vi "Login Window Control.vi"() -> ()   [LabVIEW 2015]
uses:
  <vilib>/Utility/miscctls.llb/LVBoundsTypeDef.ctl
  <vilib>/Utility/miscctls.llb/LVPositionTypeDef.ctl
  EnumEstado.ctl
  Application/Type Ref. Notificacion Eventos.ctl
  Control 2.ctl
  Control 1.ctl
panel:
  in  "Stop Button":bool
  out "Tab Control 2":enum32{"MENU"}(tab)
  out "String":string
  in  "1":T1
  in  "Password":string
  in  "2":T1
  in  "3":T1
  in  "4":T1
  in  "5":T1
  in  "6":T1
  in  "7":T1
  in  "8":T1
  in  "9":T1
  in  "Log in":T1
  in  "Borrar":T1
  in  "Clear":T1
  out "Tab Control":T2(tab)
  in  "Tab1_Button_Temperatura_ambiente":bool
  in  "Tab1_Button_Temperatura_superficie":bool
  in  "Tab1_Button_Sinoptico":bool
  in  "logout":bool
  in  "Tab1_Button_Humedad":bool
  in  "Tab1_Button_Potencia":bool
  in  "Tab1_Button_Radiacion":bool
  out "Flujo_Bypass":bool
  out "Flujo_Load":bool
  out "Flujo_Bat_descarga":bool
  out "Flujo_Bat_carg":bool
  out "Flujo_Gen":bool
  out "Flujo_Panel":bool
  out "String 11":string
  out "String 10":string
  out "String 9":string
  out "String 8":string
  in  "Tab1_volver_sinoptico":bool
  out "Falla monofásica":bool caption="Falla \nmonofásica"
  out "Algun mal funcionamiento \nen el SGH":bool caption="Algun mal funcionamiento\nen el SGH"
  out "Alta temperatura\n en gabinete":bool caption="Alta temperatura en \ngabinete"
  out "Falla trifásica":bool caption="Falla\ntrifásica"
  out "Falla en módulo":bool
  out "valor_panel":dbl
  out "valor_carga":dbl
  out "valor_generador":dbl
  out "ÚLTIMA MEDICIÓN DEL\n G. DIESEL":timestamp
  out "ÚLTIMA MEDICIÓN DEL \nINVERSOR":timestamp
  out "valor_bateria":dbl
  out "Falla nivel de batería alta":bool caption="Falla nivel \nde\nbatería alta"
  out "Nivel de batería baja":bool caption="Nivel de\nbatería baja"
  out "Ring_Panel":u16(ring)
  out "Ring_Nivel_bat":u16(ring)
  out "Ring_Gen":u16(ring)
  out "Ring_Load":u16(ring)
  out "String 7":string
  out "Ring_Inversor":u16(ring)
  out "String 2":string
  in  "Radiacion Tab 1":bool
  in  "Tab1_volver_radiacion":bool
  out "Radiacion solar global":cluster{timestamp[], dbl[]}(graph)
  in  "Temperatura Tab 1":bool
  in  "Tab1_volver_tempambiente":bool
  out "XY Graph Temperatura":cluster{timestamp[], dbl[]}(graph)
  out "String 3":string
  in  "Tab1_volver_humedad":bool
  in  "Humedad Relativa Tab 1":bool
  out "XY Humedad Relativa":T3
  out "String 4":string
  in  "Temperatura de Panel Tab 1":bool
  in  "Tab1_volver_tempsuper":bool
  out "XY Graph Temperatura de Panel":cluster{timestamp[], dbl[]}(graph)
  out "String 5":string
  in  "Tab1_volver_potencia":bool
  in  "Pot_load_S Tab 1":bool
  in  "Pot_load_R Tab 1":bool
  in  "Potencia Panel Tab 1":bool
  in  "Pot_load_T Tab 1":bool
  in  "Pot_bat. Tab 1":bool
  in  "Pot_gen Tab 1":bool
  out "XY Graph Potencia":cluster{timestamp[], dbl[]}(graph)
  out "String 6":string
  # "SISTEMA DE MONITOREO PLANTA FOTOVOLTAICA \nMAYOR PABLO LAGERENZA"
  # "ACCESO"
  # "POTENCIA"
  # "ALMACENAMIENTO"
  # "SALIDA"
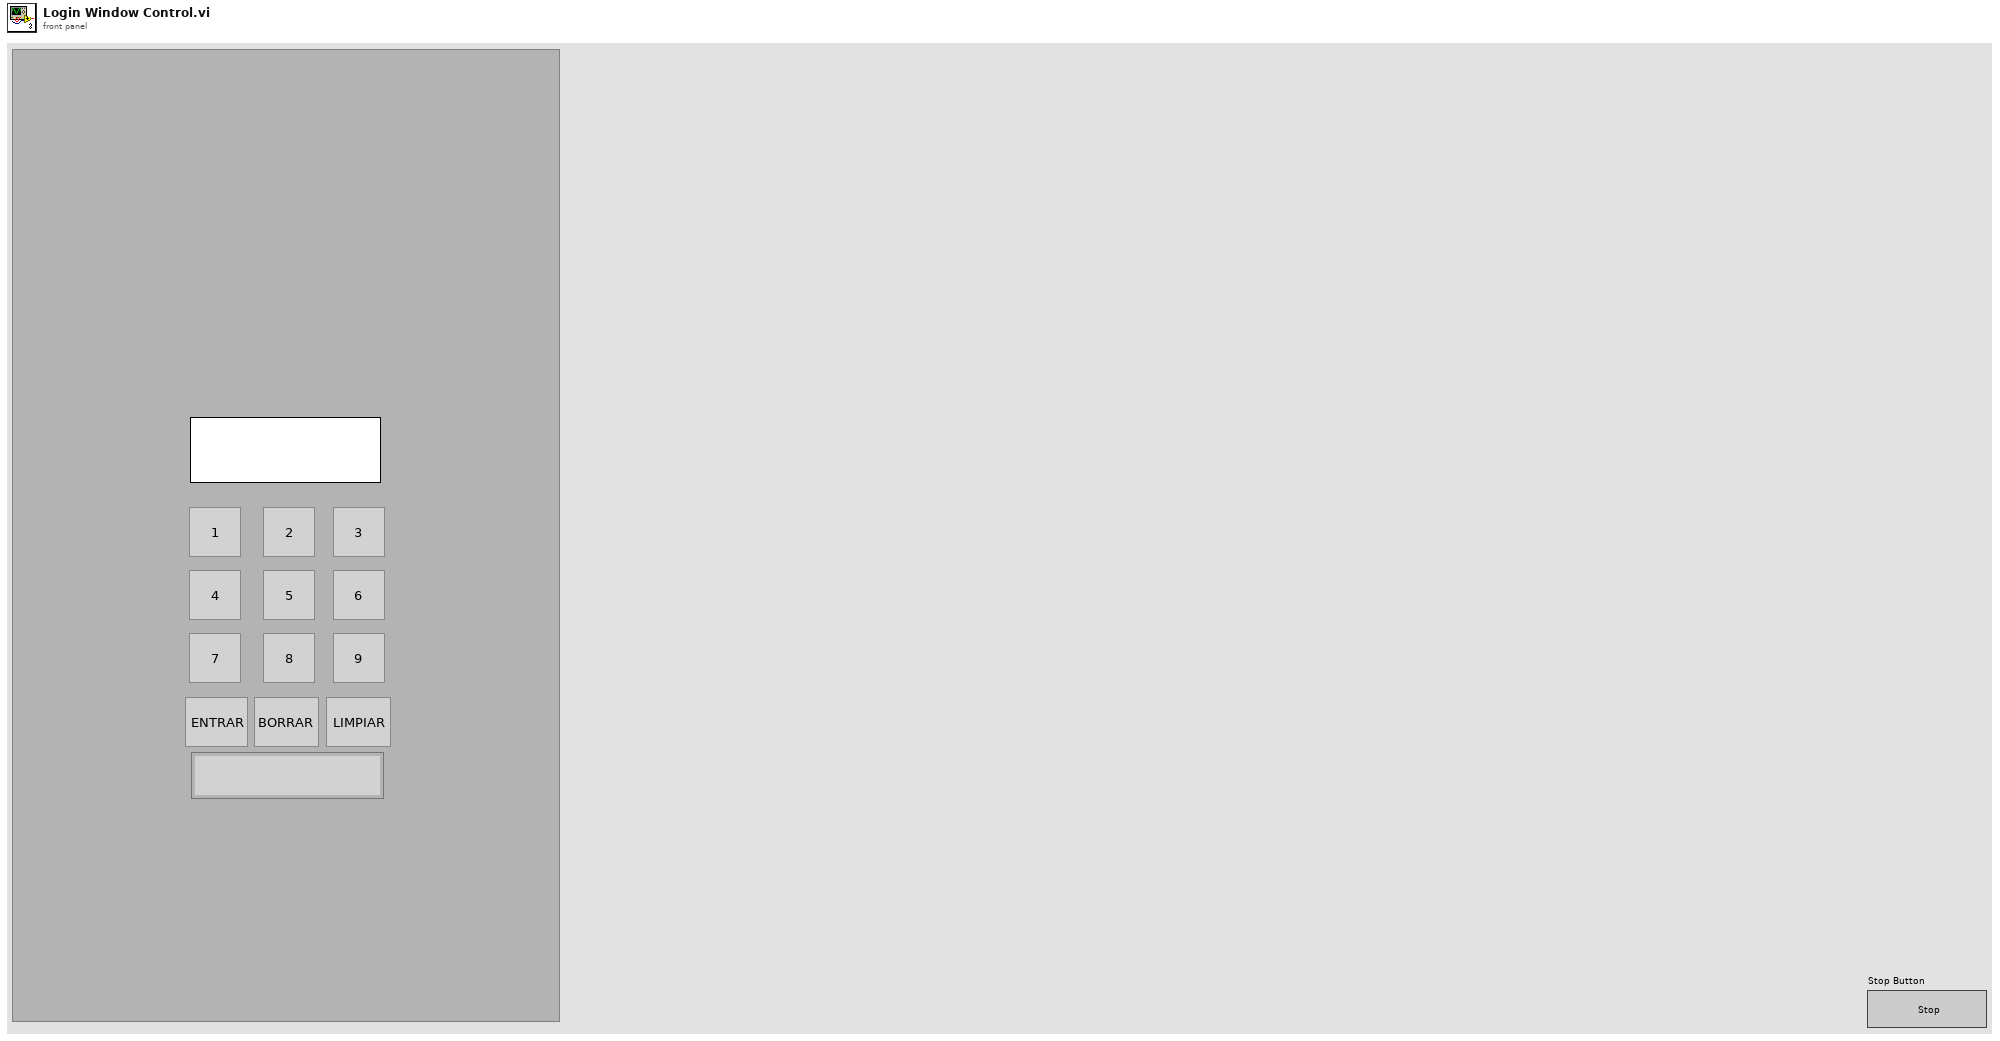
[diagram p1: front panel]
types:
  T1 = typedef "Control 2.ctl" = bool
  T2 = enum32{"MENU", "CUADRO SINOPTICO", "RADIACION SOLAR", "TEMPERATURA", "HUMEDAD RELATIVA", "TEMPERATURA DE SUPERFICIE", "POTENCIA"}
  T3 = typedef "Control 1.ctl" = cluster{timestamp[], dbl[]}
  T4 = typedef "LVPositionTypeDef.ctl" = cluster{"Left":i32, "Top":i32}
  T5 = typedef "LVBoundsTypeDef.ctl" = cluster{"Width":u32, "Height":u32}
  T6 = cluster{"queueM1 out":refnum<queue>, "queueM2 out":refnum<queue>, "queueM3 out":refnum<queue>}
  T7 = typedef "EnumEstado.ctl" = enum16{"Stop", "Iniciado", "Log In", "Log Out", "Escribir", "Leer Radiacion", "Leer Temp", "Leer Humed Relat", "Leer Temp del Panel", "Leer Pot Panel", "Leer Pot Fase R", "Leer Pot Fase  S", "Leer PotFase T", "Leer Nivel Bat", "Leer Pot Generador"}
  T8 = typedef "Type Ref. Notificacion Eventos.ctl" = enum32{"MENU", "CUADRO SINOPTICO", "RADIACION SOLAR", "TEMPERATURA", "HUMEDAD RELATIVA", "TEMPERATURA DE SUPERFICIE", "POTENCIA"}
  T9 = typedef "Semaphore RefNum" = refnum<k1>
  T10 = enum16{"open", "replace", "create", "open or create", "replace or create", "replace or create with confirmation"}
  T11 = cluster{"tdms control out":refnum<k34>, "tdms historial out":refnum<k34>, "tdms sinc out":refnum<k34>}
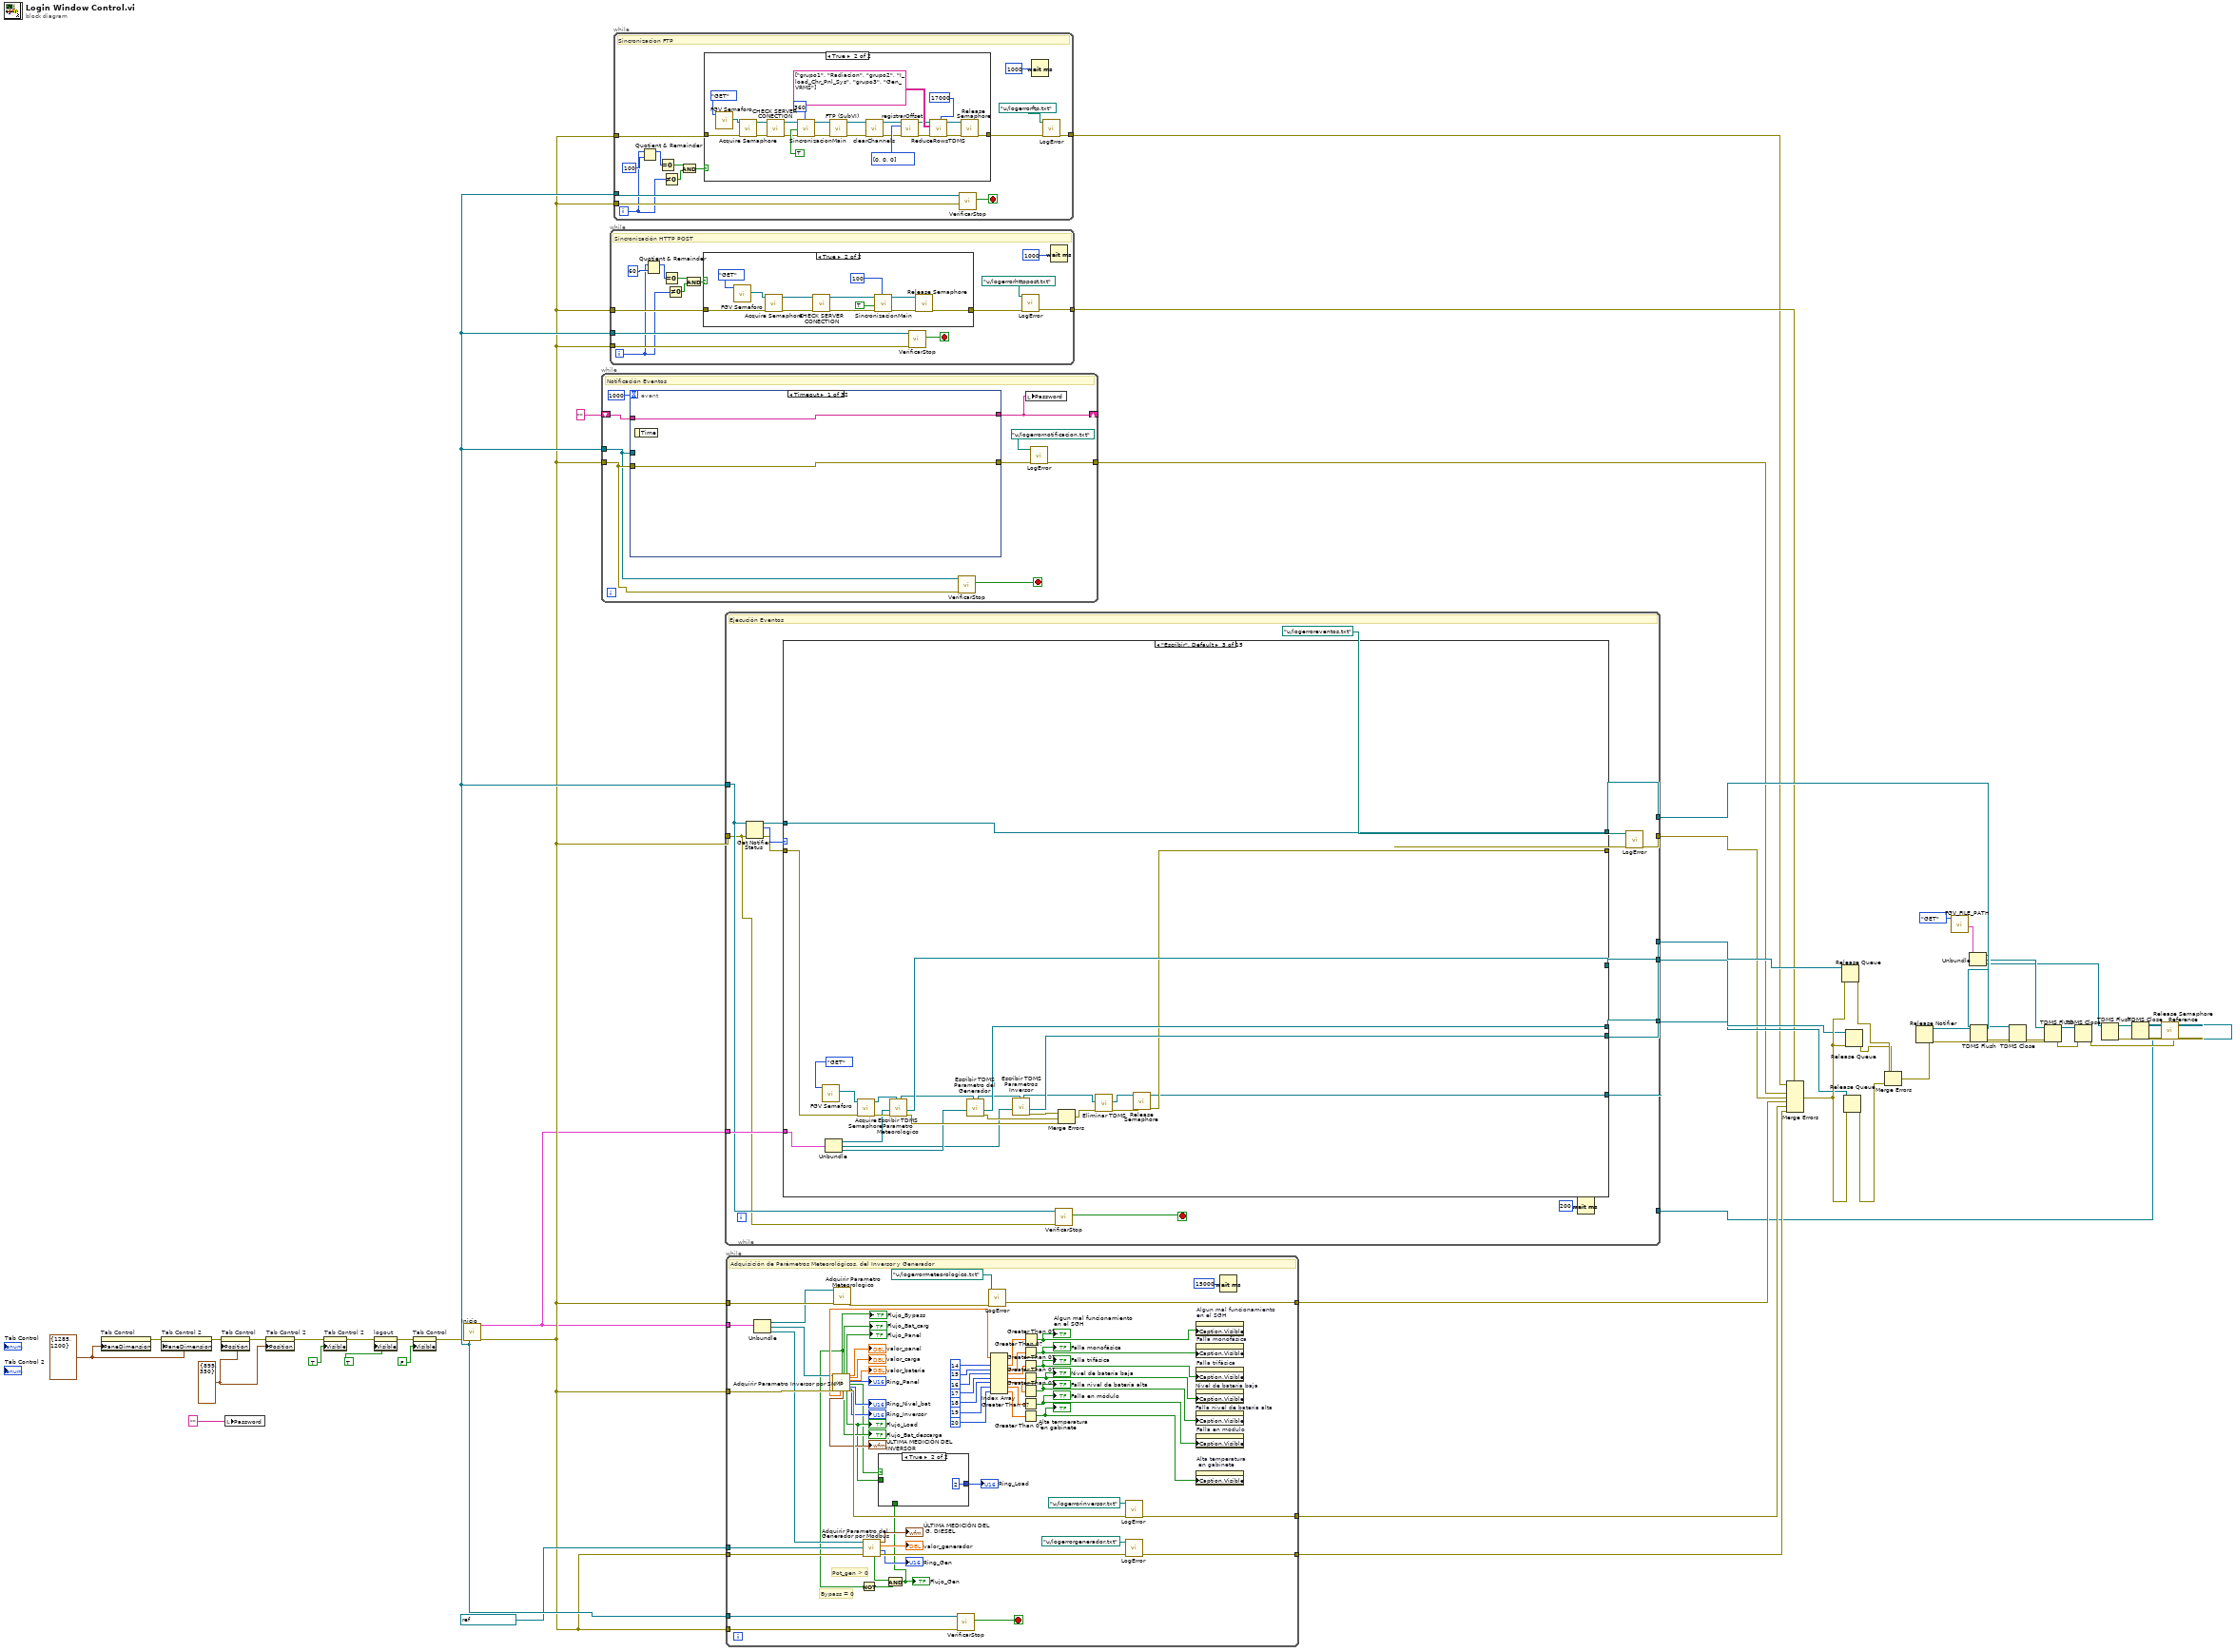
[diagram p0: block diagram]
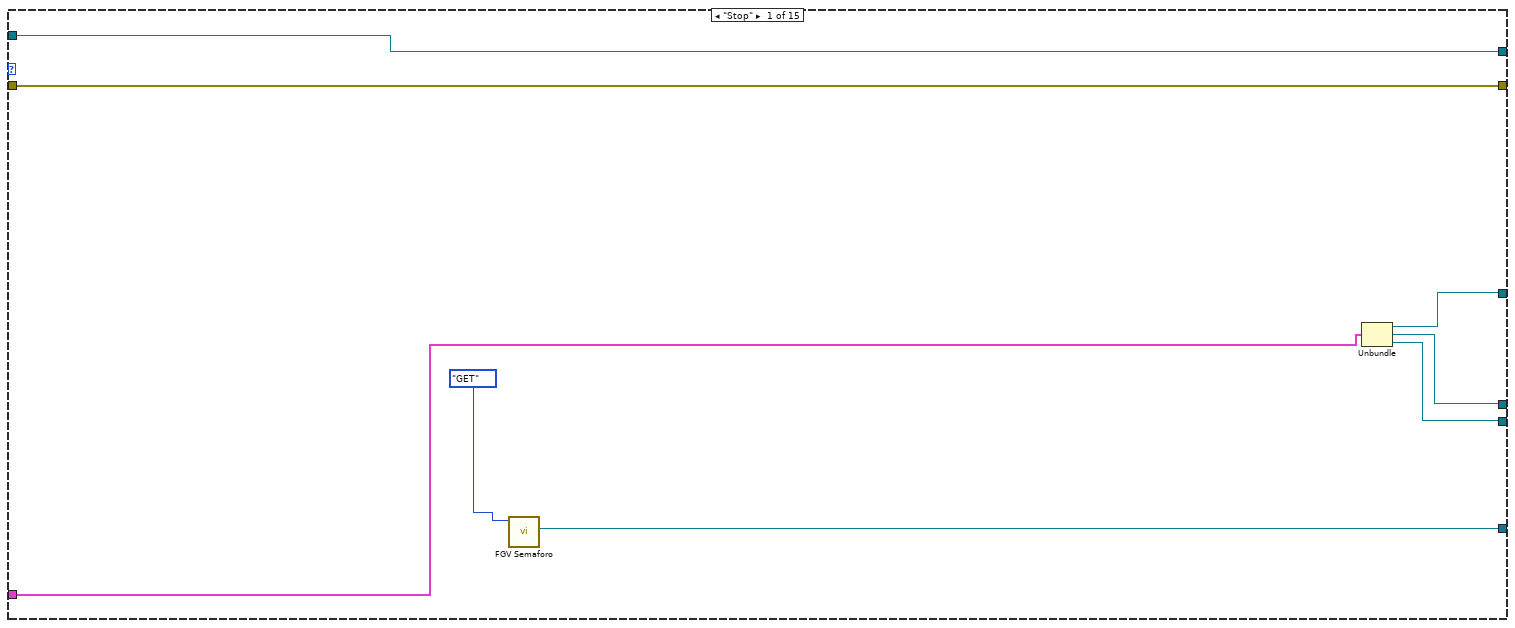
[diagram p4: hidden frame]
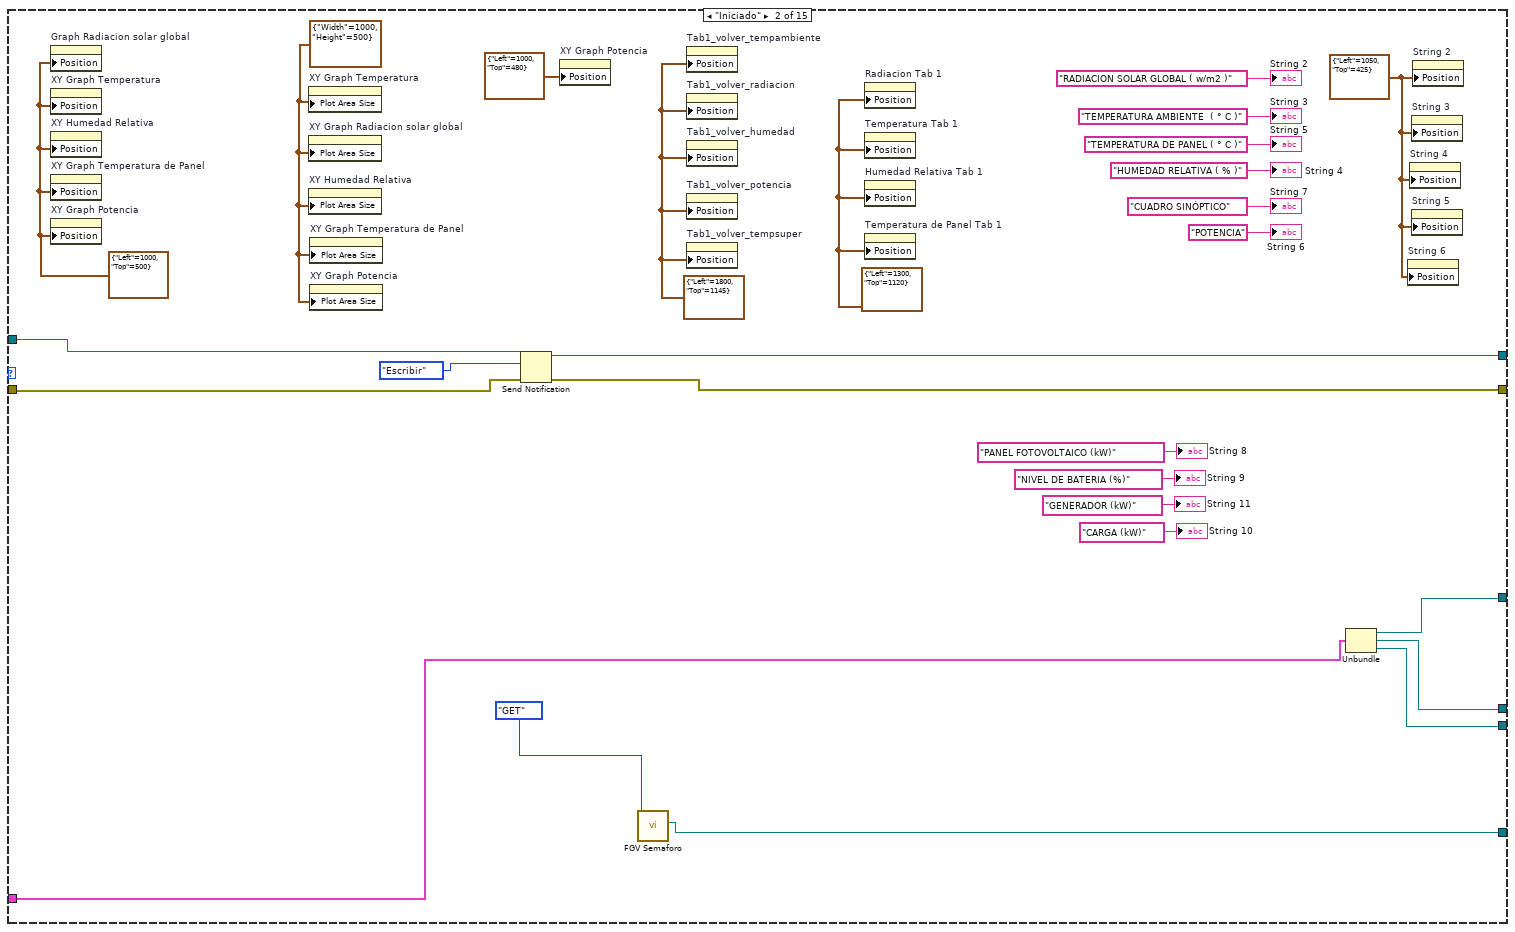
[diagram p5: hidden frame]
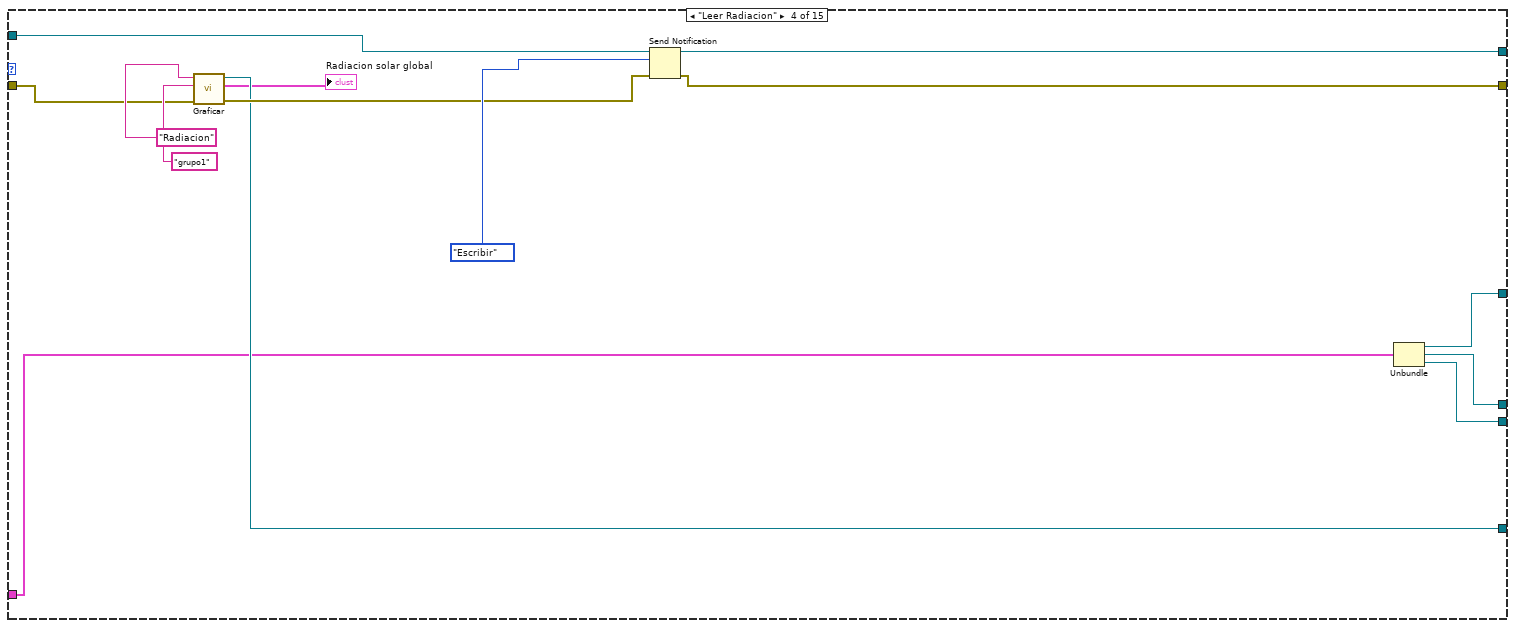
[diagram p6: hidden frame]
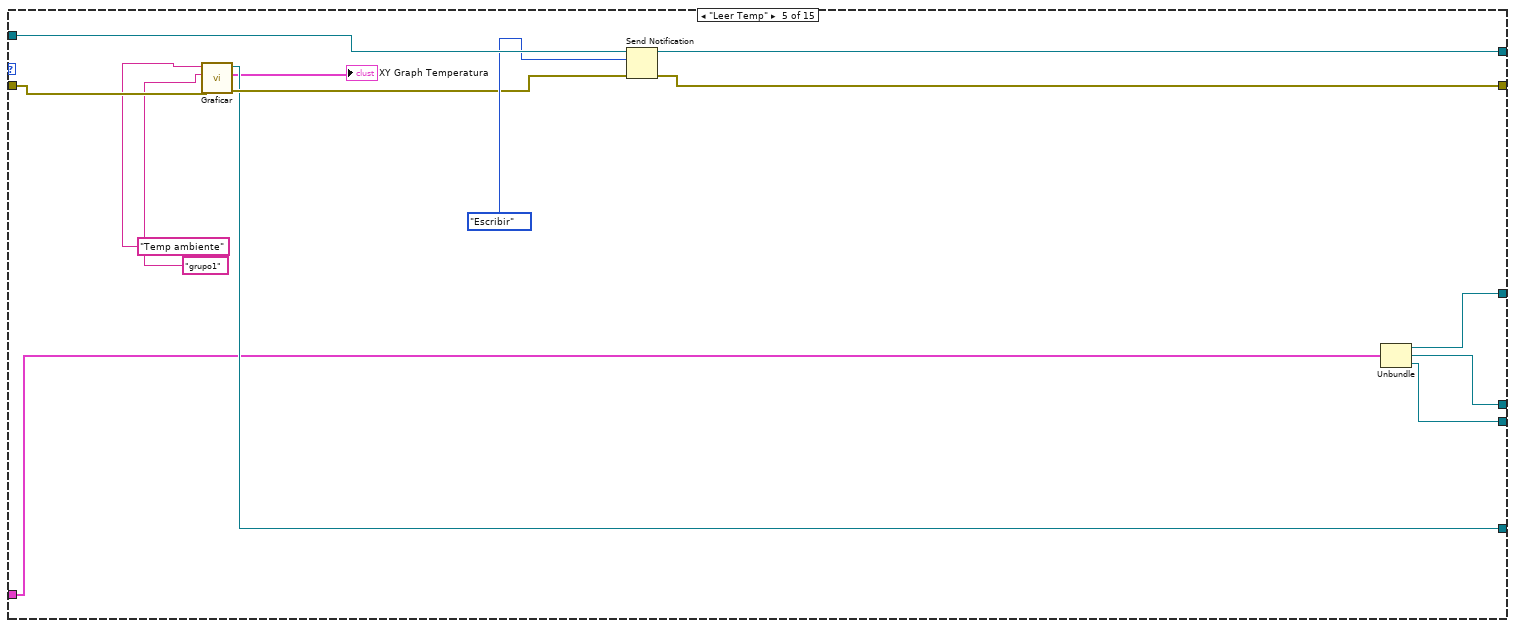
[diagram p7: hidden frame]
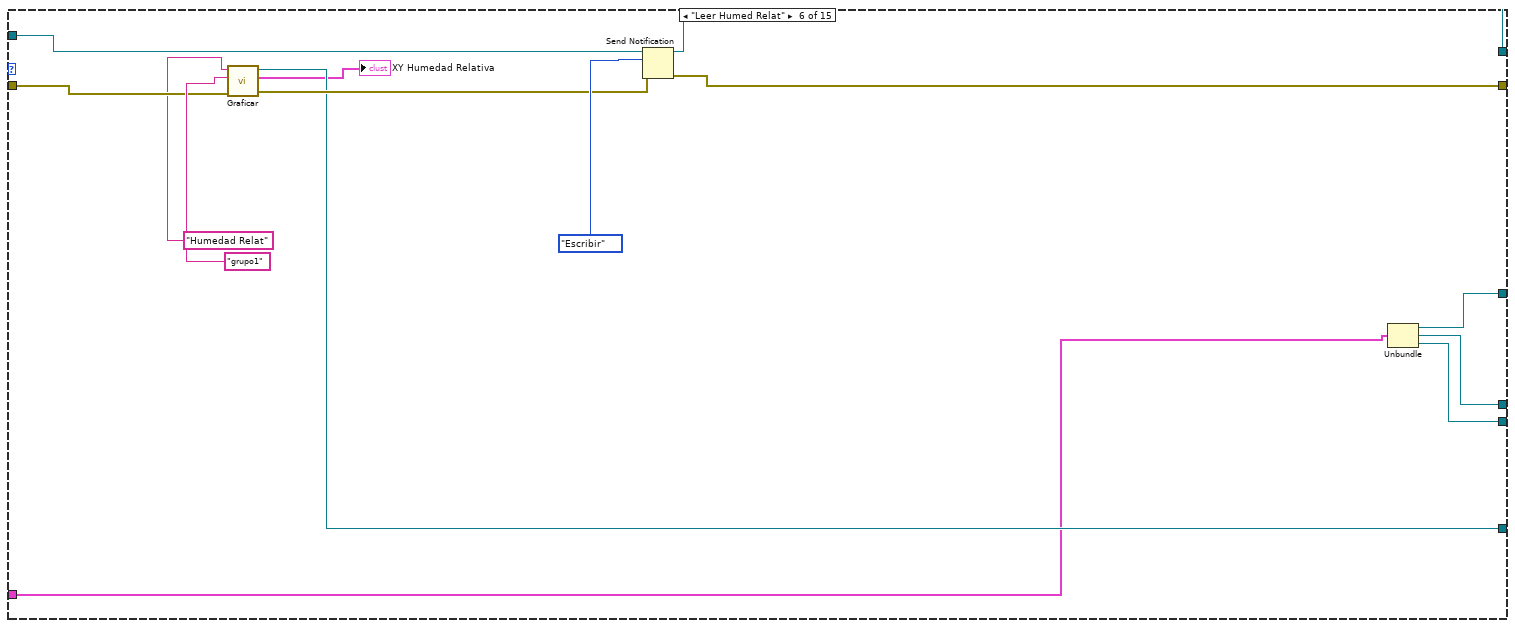
[diagram p8: hidden frame]
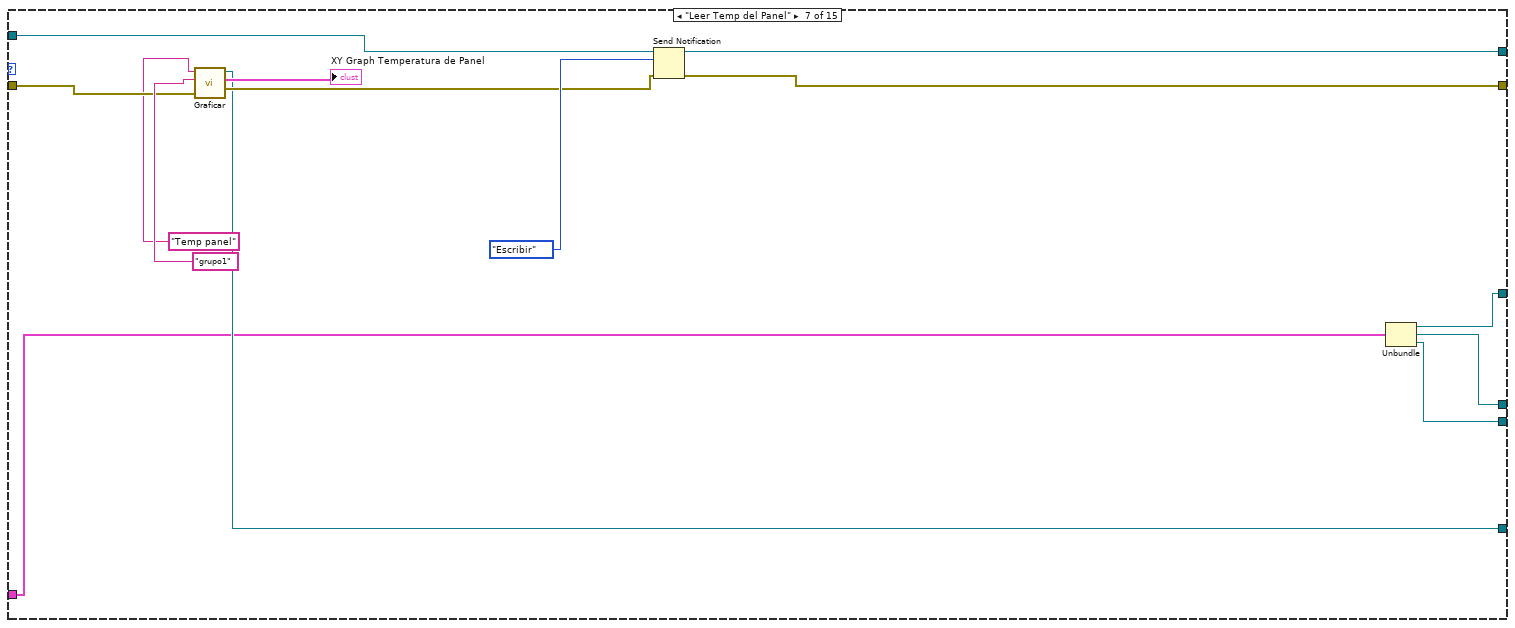
[diagram p9: hidden frame]
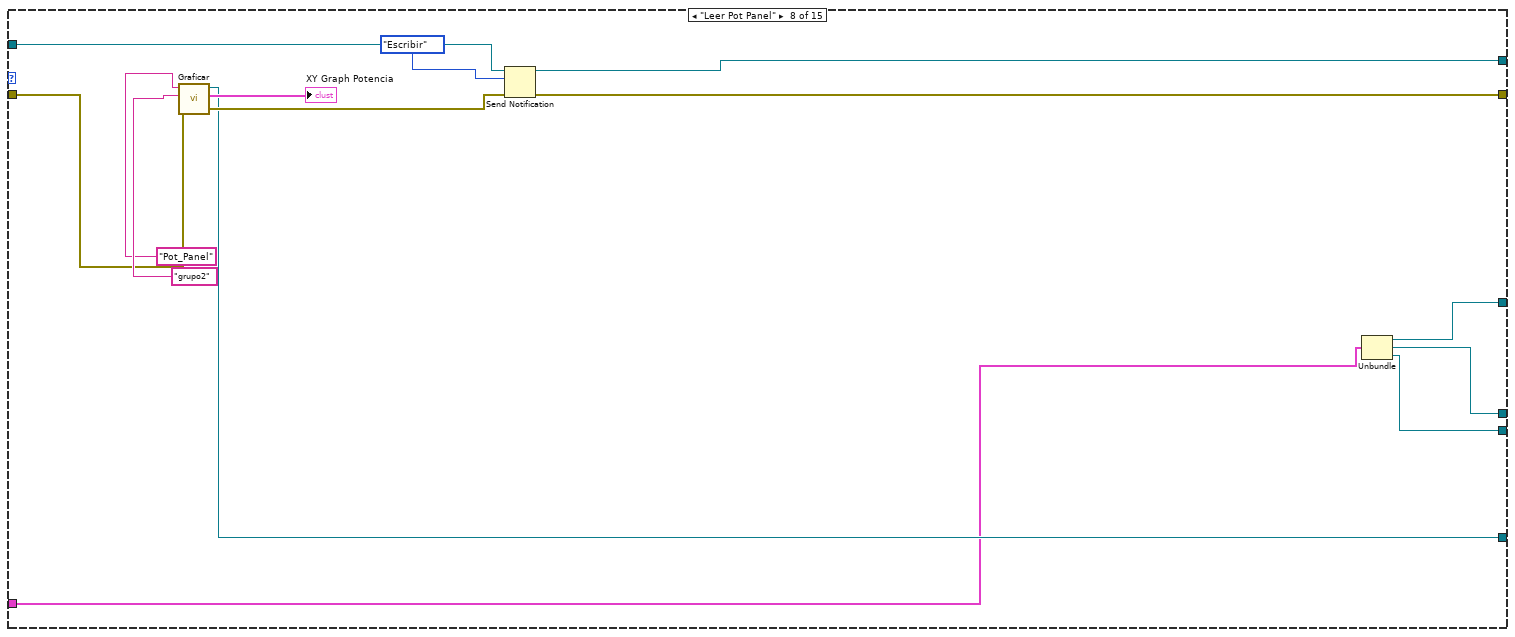
[diagram p10: hidden frame]
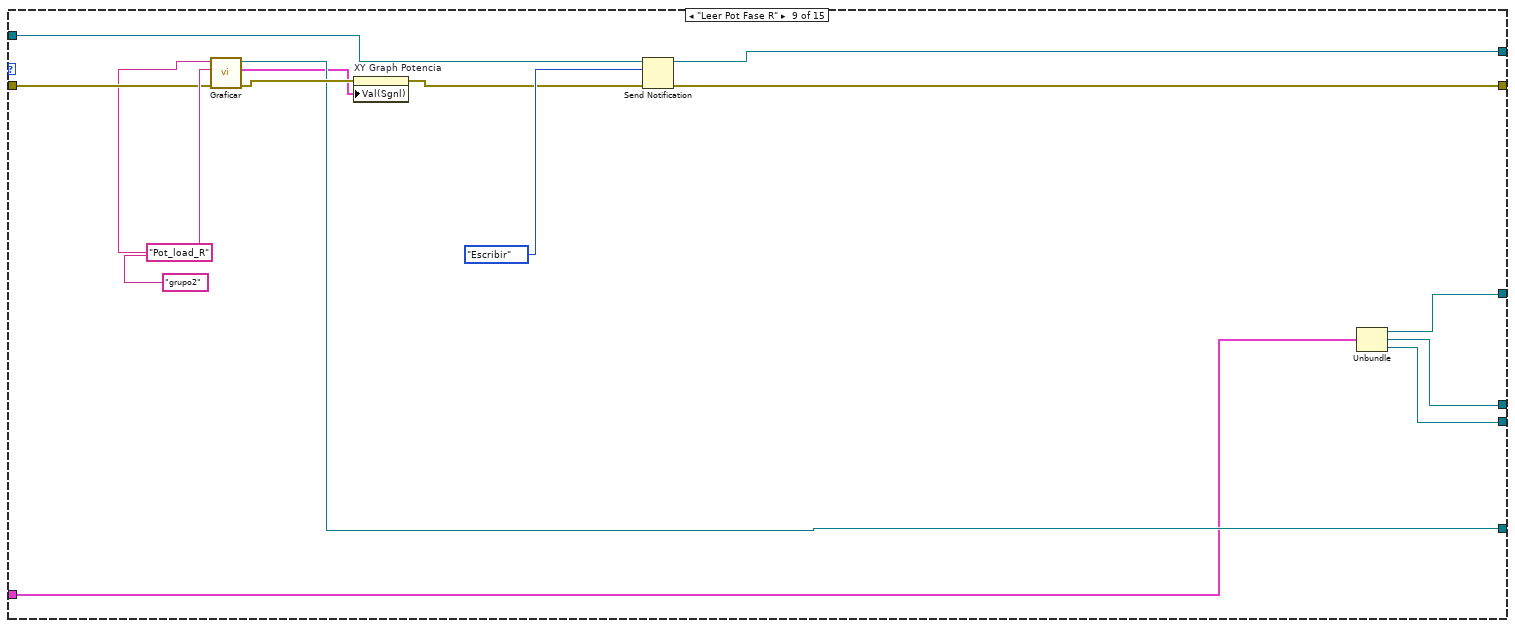
[diagram p11: hidden frame]
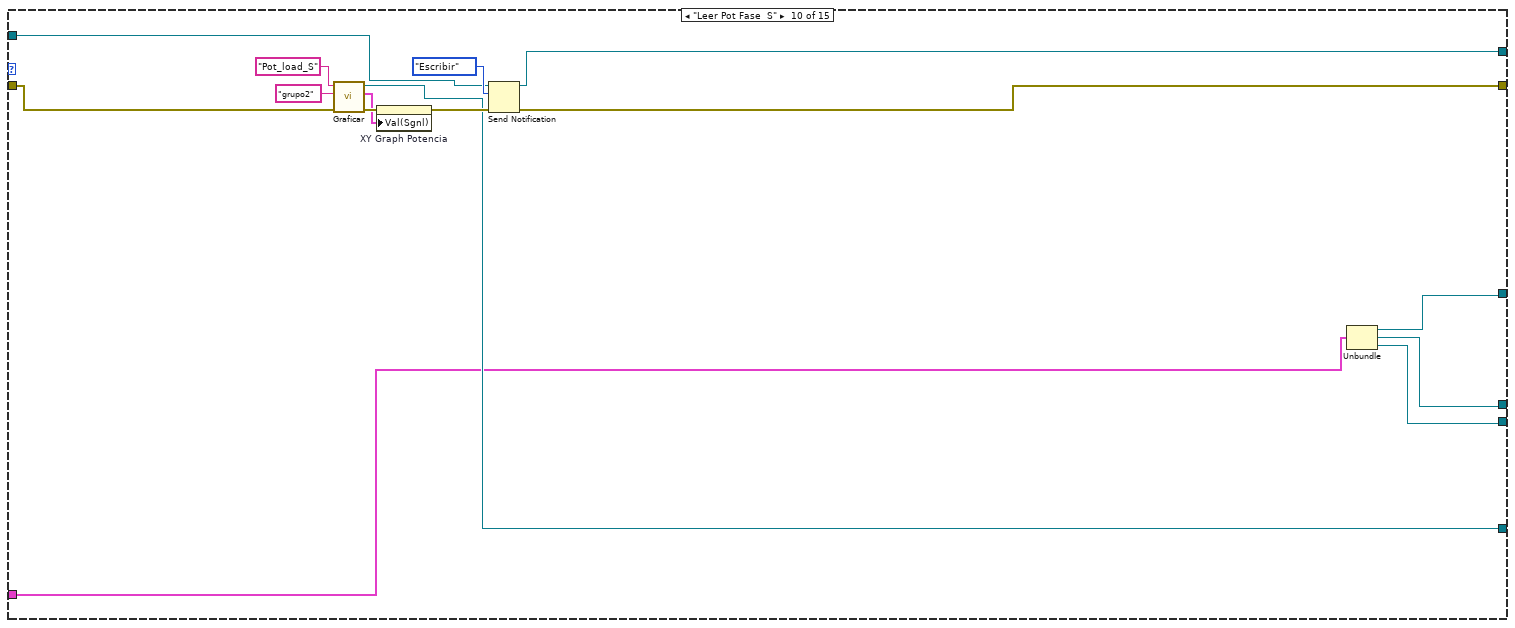
[diagram p12: hidden frame]
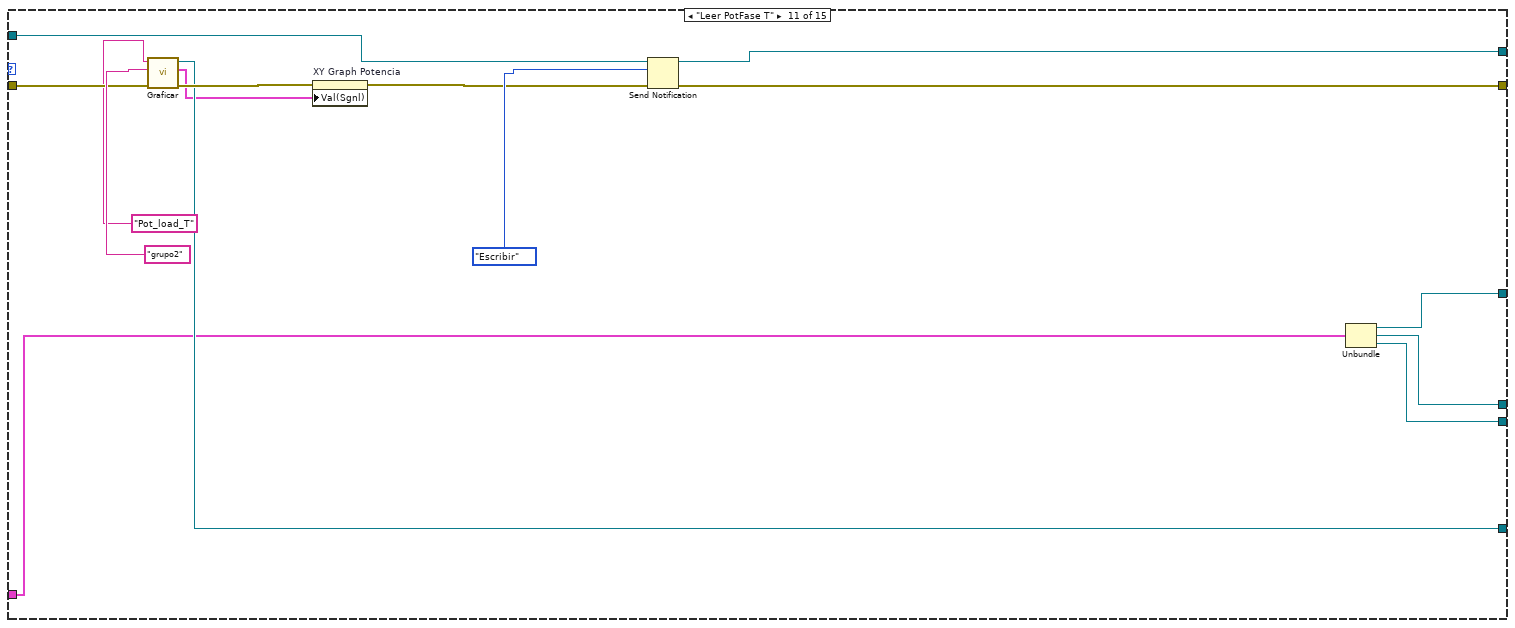
[diagram p13: hidden frame]
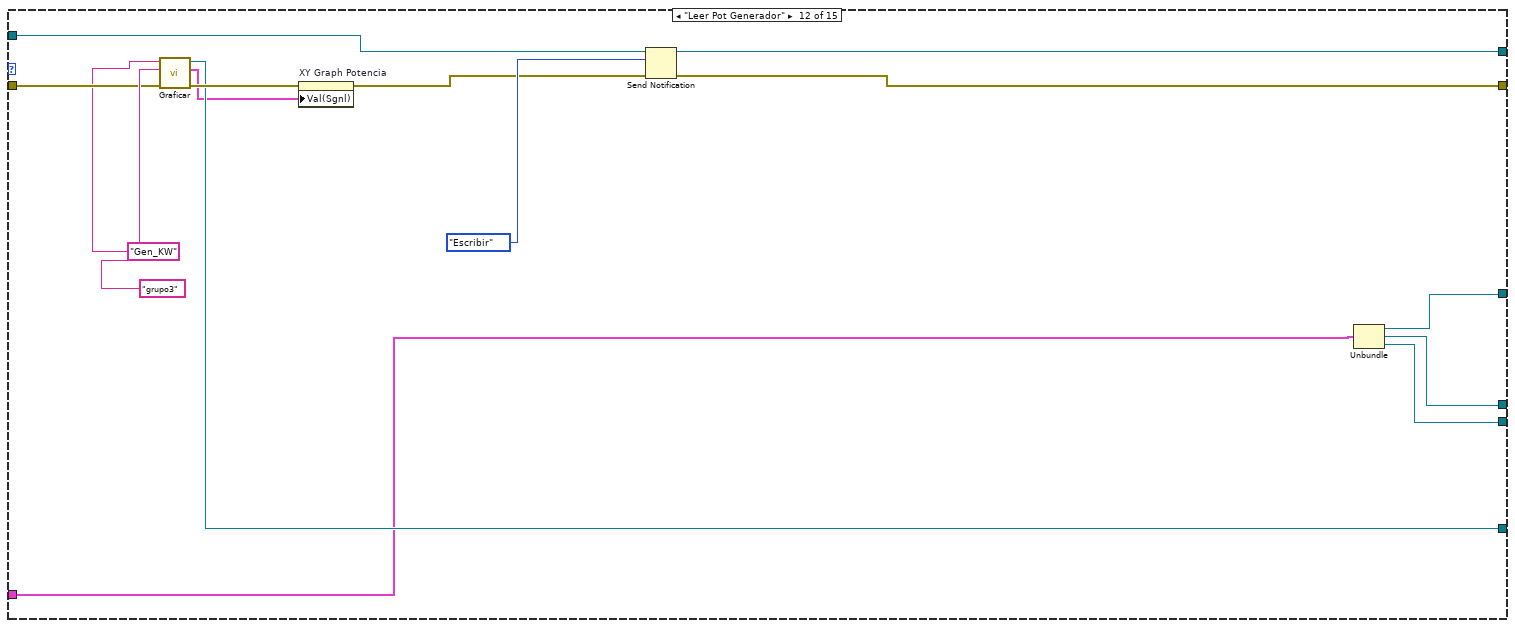
[diagram p14: hidden frame]
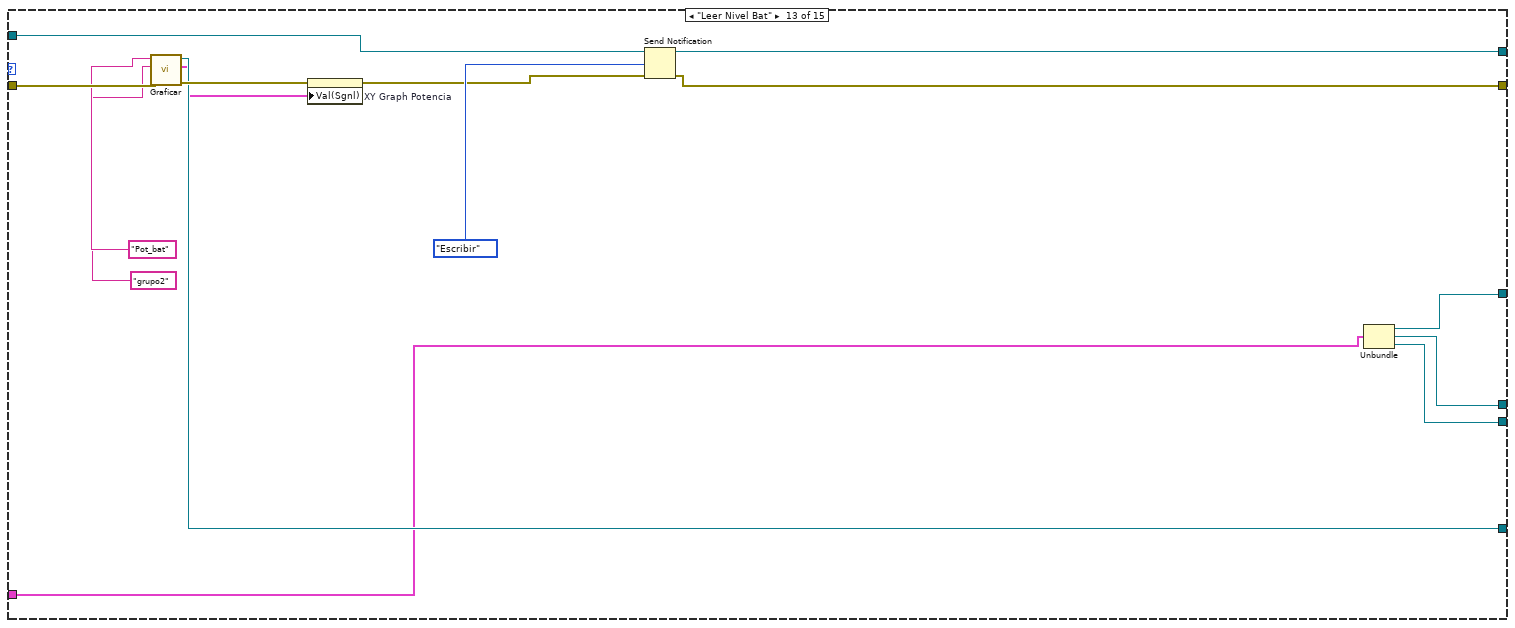
[diagram p15: hidden frame]
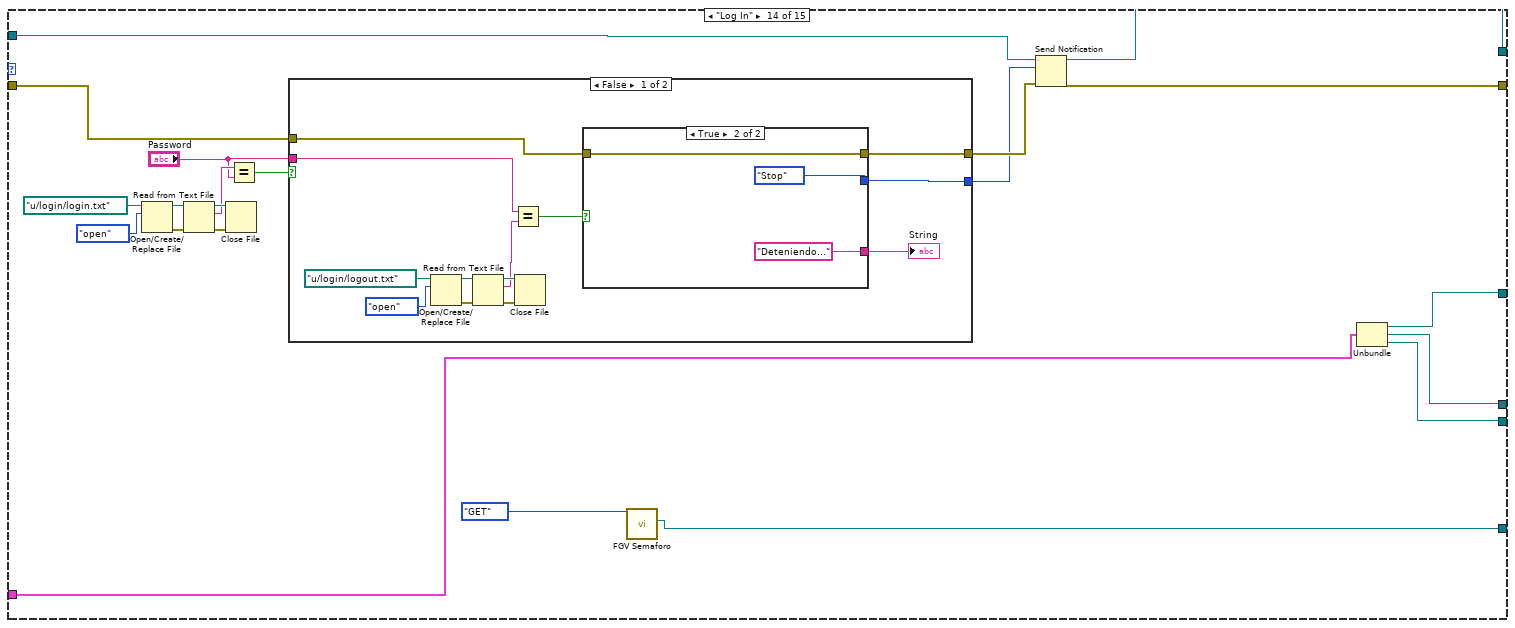
[diagram p16: hidden frame]
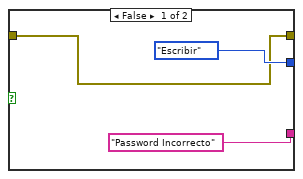
[diagram p17: hidden frame]
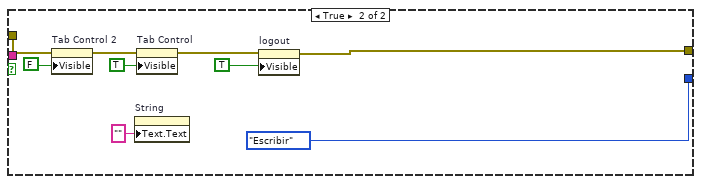
[diagram p18: hidden frame]
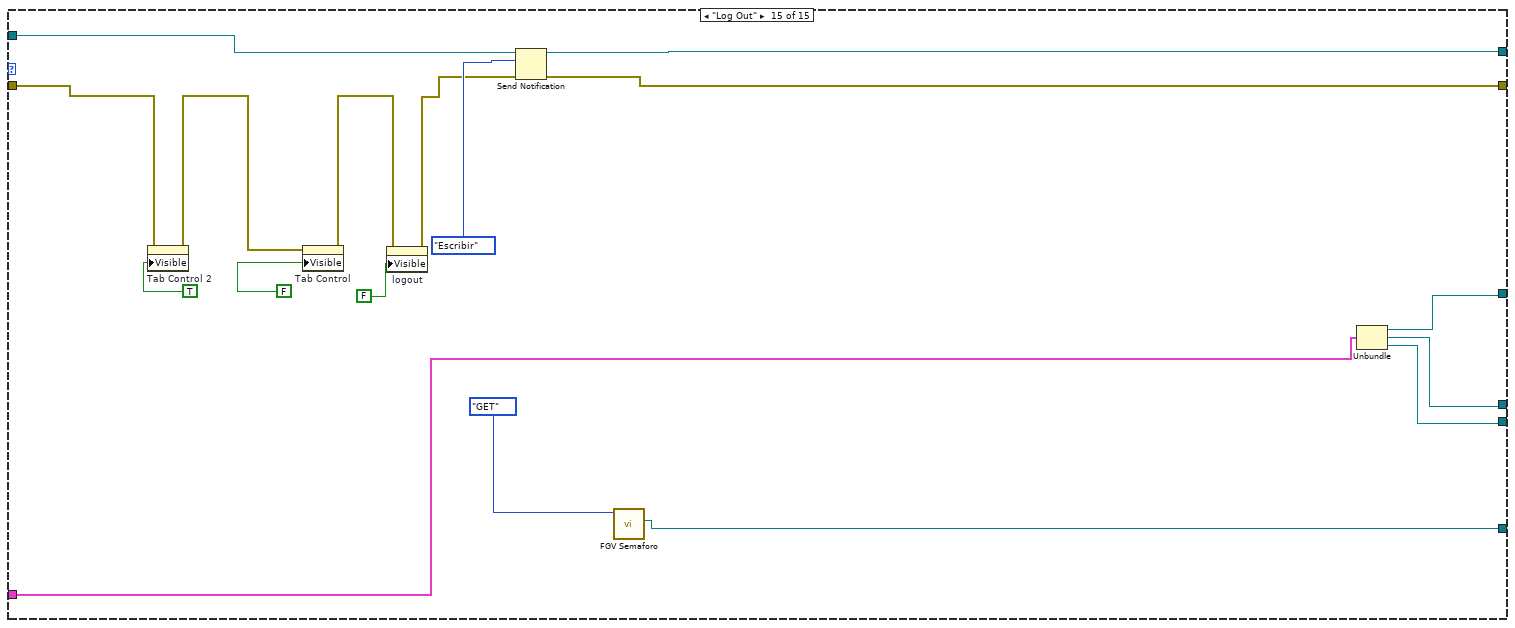
[diagram p19: hidden frame]
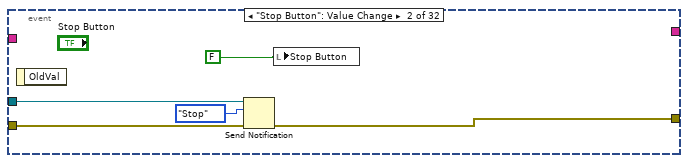
[diagram p20: hidden frame]
diagram:
  w22 = T4 {"Left"=895, "Top"=350} ("Position")
  w17 = T5 {"Width"=1285, "Height"=1200} ("Tab Control Pane Dimension")
  n1 = property on="Tab Control" class="TabCtl (strict)"("PaneDimension"=w17) -> (error out=w18:errorcluster)  [unwired: 2 in, 1 out]
  n2 = property on="Tab Control 2" class="TabCtl (strict)"(error in=w18, "PaneDimension"=w17) -> (error out=w19:errorcluster)  [unwired: 1 in, 1 out]
  n3 = property on="Tab Control" class="TabCtl (strict)"(error in=w19, "Position"=w22) -> (error out=w23:errorcluster)  [unwired: 1 in, 1 out]
  n4 = local write "Password"("" ("Password")) -> ()
  n5 = property on="Tab Control 2" class="TabCtl (strict)"(error in=w23, "Position"=w22) -> (error out=w20:errorcluster)  [unwired: 1 in, 1 out]
  n6 = property on="Tab Control 2" class="TabCtl (strict)"(error in=w20, "Visible"=TRUE) -> (error out=w16:errorcluster)  [unwired: 1 in, 1 out]
  n7 = property on="logout" class="Bool (strict)"(error in=w16, "Visible"=TRUE) -> (error out=w15:errorcluster)  [unwired: 1 in, 1 out]
  n8 = property on="Tab Control" class="TabCtl (strict)"(error in=w15, "Visible"=FALSE) -> (error out=w12:errorcluster)  [unwired: 1 in, 1 out]
  n9 = call "Inicio.vi"("error in"=w12) -> ("Cluster"=w11:T6, "notifier out"=w31:refnum<notifier>, "error out"=w26:errorcluster)  [unwired: 12 in]
  n10 = while {
    shift-right: [w58] -> _
    shift-left: "" -> [w59]
    tunnel: w31 -> [w52]
    tunnel: [w56] -> w36
    tunnel: w26 -> [w53]
    stop <- w54 stop-if-true
    # "Notificación Eventos"
    n11 = event shown="[0] Timeout" {
      selector: _ -> [_ _ _ _ _ _ _ _ _ _ _ _ _ _ _ _ _ _ _ _ _ _ _ _ _ _ _ _ _ _ _ _]
      dyn-events: _ -> [_ _ _ _ _ _ _ _ _ _ _ _ _ _ _ _ _ _ _ _ _ _ _ _ _ _ _ _ _ _ _ _]
      timeout: 1000 -> [_ _ _ _ _ _ _ _ _ _ _ _ _ _ _ _ _ _ _ _ _ _ _ _ _ _ _ _ _ _ _ _]
      tunnel: [w61 _ w69 w75 _ _ _ _ _ _ _ _ _ _ _ w124 _ _ _ _ _ _ _ "" w151 w155 w159 w163 w167 w171 w175 w179] -> w58
      tunnel: w59 -> [w61 _ w67 w74 _ _ _ _ _ _ _ _ _ _ _ w124 _ _ _ _ _ _ _ _ w150 w153 w157 w161 w165 w169 w173 w177]
      tunnel: w52 -> [_ w65 _ _ _ w87 w90 w94 w97 w102 w106 w110 w114 w118 w122 w127 _ _ _ _ _ _ w143 _ _ _ _ _ _ _ _ _]
      tunnel: w53 -> [w60 w64 _ _ _ w84 w89 w93 w96 w101 w105 w109 w113 w117 w121 w126 w130 w132 w134 w136 w138 w140 w142 w146 w148 w152 w156 w160 w164 w168 w172 w176]
      tunnel: [w60 w63 _ _ _ w85 w88 w92 w98 w100 w104 w108 w112 w116 w120 w125 w130 w132 w134 w136 w138 w140 w141 w146 w148 w152 w156 w160 w164 w168 w172 w176] -> w57
      event Timeout {
        n12 = event-data() -> ()  [unwired: 1 in, 1 out]
      }
      event "Stop Button": Value Change {
        n13 = event-data() -> ()  [unwired: 1 in, 1 out]
        n14 = Send Notification(notification=EnumEstado."Stop", notifier=w65, error in (no error)=w64) -> (error out=w63:errorcluster)  [unwired: 1 out]
        n15 = local write "Stop Button"(FALSE ("Stop Button")) -> ()
      }
      event Value Change {
        n16 = event-data() -> ()  [unwired: 1 in, 1 out]
        n17 = Concatenate Strings(w67, "1") -> (w69:string)
      }
      event Value Change {
        n18 = event-data() -> ()  [unwired: 1 in, 1 out]
        n19 = String Length(string=w74) -> (length=w73:i32)
        n20 = Less Or Equal?(x=w73, y=1) -> (x <= y?=w71:bool)
        n21 = case shown="True" w71 {
          tunnel: [w78 ""] -> w75
          tunnel: w74 -> [w76 _]
          frame False {
            n22 = Decimal String To Number(string=w76) -> (number=w80:i32)  [unwired: 2 in, 1 out]
            n23 = Quotient & Remainder(x=w80, y=10) -> (floor(x/y)=w77:i32)  [unwired: 1 out]
            n24 = Number To Decimal String(number=w77) -> (decimal integer string=w78:string)  [unwired: 1 in]
          }
          frame True {
          }
        }
        n25 = property on="String" class="Str"("Text.Text"="") -> ()  [unwired: 2 in, 2 out]
      }
      event "Tab1_volver_tempambiente", "Tab1_volver_tempsuper", "Tab1_volver_humedad", "Tab1_volver_potencia", "Tab1_volver_radiacion", "Tab1_volver_sinoptico": Value Change {
        w82 = cluster{timestamp[], dbl[]} {[], []} ("Radiacion solar global")
        n26 = event-data() -> ()  [unwired: 1 in, 6 out]
        n27 = local write "Tab Control"(Type_Ref._Notificacion_Eventos."MENU" ("Tab Control")) -> ()
        n28 = property on="Radiacion solar global" class="XYGraph (strict)"("Value"=w82) -> ()  [unwired: 2 in, 2 out]
        n29 = property on="XY Graph Temperatura" class="XYGraph (strict)"("Value"=w82) -> ()  [unwired: 2 in, 2 out]
        n30 = property on="XY Humedad Relativa" class="XYGraph (strict)"("Value"=w82) -> ()  [unwired: 2 in, 2 out]
        n31 = property on="XY Graph Temperatura de Panel" class="XYGraph (strict)"("Value"=w82) -> ()  [unwired: 2 in, 2 out]
        n32 = property on="XY Graph Potencia" class="XYGraph (strict)"("Value"=w82) -> ()  [unwired: 2 in, 2 out]
      }
      event "Radiacion Tab 1": Value Change {
        n33 = event-data() -> ()  [unwired: 1 in, 6 out]
        n34 = Send Notification(notification=EnumEstado."Leer Radiacion", notifier=w87, error in (no error)=w84) -> (error out=w85:errorcluster)  [unwired: 1 out]
      }
      event "Temperatura Tab 1": Value Change {
        n35 = event-data() -> ()  [unwired: 1 in, 1 out]
        n36 = Send Notification(notification=EnumEstado."Leer Temp", notifier=w90, error in (no error)=w89) -> (error out=w88:errorcluster)  [unwired: 1 out]
      }
      event "Humedad Relativa Tab 1": Value Change {
        n37 = event-data() -> ()  [unwired: 1 in, 6 out]
        n38 = Send Notification(notification=EnumEstado."Leer Humed Relat", notifier=w94, error in (no error)=w93) -> (error out=w92:errorcluster)  [unwired: 1 out]
      }
      event "Temperatura de Panel Tab 1": Value Change {
        n39 = event-data() -> ()  [unwired: 1 in, 6 out]
        n40 = Send Notification(notification=EnumEstado."Leer Temp del Panel", notifier=w97, error in (no error)=w96) -> (error out=w98:errorcluster)  [unwired: 1 out]
      }
      event "Potencia Panel Tab 1": Value Change {
        n41 = event-data() -> ()  [unwired: 1 in, 1 out]
        n42 = Send Notification(notification=EnumEstado."Leer Pot Panel", notifier=w102, error in (no error)=w101) -> (error out=w100:errorcluster)  [unwired: 1 out]
      }
      event "Pot_load_R Tab 1": Value Change {
        n43 = event-data() -> ()  [unwired: 1 in, 1 out]
        n44 = Send Notification(notification=EnumEstado."Leer Pot Fase R", notifier=w106, error in (no error)=w105) -> (error out=w104:errorcluster)  [unwired: 1 out]
      }
      event "Pot_load_S Tab 1": Value Change {
        n45 = event-data() -> ()  [unwired: 1 in, 1 out]
        n46 = Send Notification(notification=EnumEstado."Leer Pot Fase  S", notifier=w110, error in (no error)=w109) -> (error out=w108:errorcluster)  [unwired: 1 out]
      }
      event "Pot_load_T Tab 1": Value Change {
        n47 = event-data() -> ()  [unwired: 1 in, 1 out]
        n48 = Send Notification(notification=EnumEstado."Leer PotFase T", notifier=w114, error in (no error)=w113) -> (error out=w112:errorcluster)  [unwired: 1 out]
      }
      event "Pot_bat. Tab 1": Value Change {
        n49 = event-data() -> ()  [unwired: 1 in, 1 out]
        n50 = Send Notification(notification=EnumEstado."Leer Nivel Bat", notifier=w118, error in (no error)=w117) -> (error out=w116:errorcluster)  [unwired: 1 out]
      }
      event "Pot_gen Tab 1": Value Change {
        n51 = event-data() -> ()  [unwired: 1 in, 1 out]
        n52 = Send Notification(notification=EnumEstado."Leer Pot Generador", notifier=w122, error in (no error)=w121) -> (error out=w120:errorcluster)  [unwired: 1 out]
      }
      event Value Change {
        # "Set Password"
        n53 = event-data() -> ()  [unwired: 1 in, 1 out]
        n54 = Send Notification(notification=EnumEstado."Log In", notifier=w127, error in (no error)=w126) -> (error out=w125:errorcluster)  [unwired: 1 out]
      }
      event "Tab1_Button_Temperatura_ambiente": Value Change {
        n55 = event-data() -> ()  [unwired: 1 in, 1 out]
        n56 = local write "Tab Control"(Type_Ref._Notificacion_Eventos."TEMPERATURA" ("Tab Control")) -> ()
      }
      event "Tab1_Button_Humedad": Value Change {
        n57 = event-data() -> ()  [unwired: 1 in, 1 out]
        n58 = local write "Tab Control"(Type_Ref._Notificacion_Eventos."HUMEDAD RELATIVA" ("Tab Control")) -> ()
      }
      event "Tab1_Button_Potencia": Value Change {
        n59 = event-data() -> ()  [unwired: 1 in, 1 out]
        n60 = local write "Tab Control"(Type_Ref._Notificacion_Eventos."POTENCIA" ("Tab Control")) -> ()
      }
      event "Tab1_Button_Temperatura_superficie": Value Change {
        n61 = event-data() -> ()  [unwired: 1 in, 1 out]
        n62 = local write "Tab Control"(Type_Ref._Notificacion_Eventos."TEMPERATURA DE SUPERFICIE" ("Tab Control")) -> ()
      }
      event "Tab1_Button_Radiacion": Value Change {
        n63 = event-data() -> ()  [unwired: 1 in, 1 out]
        n64 = local write "Tab Control"(Type_Ref._Notificacion_Eventos."RADIACION SOLAR" ("Tab Control")) -> ()
      }
      event "Tab1_Button_Sinoptico": Value Change {
        n65 = event-data() -> ()  [unwired: 1 in, 1 out]
        n66 = local write "Tab Control"(Type_Ref._Notificacion_Eventos."CUADRO SINOPTICO" ("Tab Control")) -> ()
      }
      event "logout": Value Change {
        n67 = event-data() -> ()  [unwired: 1 in, 6 out]
        n68 = Send Notification(notification=EnumEstado."Log Out", notifier=w143, error in (no error)=w142) -> (error out=w141:errorcluster)  [unwired: 1 out]
      }
      event Value Change {
        n69 = event-data() -> ()  [unwired: 1 in, 1 out]
        n70 = property on="String" class="Str"("Text.Text"="") -> ()  [unwired: 2 in, 2 out]
      }
      event Value Change {
        n71 = event-data() -> ()  [unwired: 1 in, 1 out]
        n72 = Concatenate Strings(w150, "2") -> (w151:string)
      }
      event Value Change {
        n73 = event-data() -> ()  [unwired: 1 in, 1 out]
        n74 = Concatenate Strings(w153, "3") -> (w155:string)
      }
      event Value Change {
        n75 = event-data() -> ()  [unwired: 1 in, 1 out]
        n76 = Concatenate Strings(w157, "4") -> (w159:string)
      }
      event Value Change {
        n77 = event-data() -> ()  [unwired: 1 in, 1 out]
        n78 = Concatenate Strings(w161, "5") -> (w163:string)
      }
      event Value Change {
        n79 = event-data() -> ()  [unwired: 1 in, 1 out]
        n80 = Concatenate Strings(w165, "6") -> (w167:string)
      }
      event Value Change {
        n81 = event-data() -> ()  [unwired: 1 in, 1 out]
        n82 = Concatenate Strings(w169, "7") -> (w171:string)
      }
      event Value Change {
        n83 = event-data() -> ()  [unwired: 1 in, 1 out]
        n84 = Concatenate Strings(w173, "8") -> (w175:string)
      }
      event Value Change {
        n85 = event-data() -> ()  [unwired: 1 in, 1 out]
        n86 = Concatenate Strings(w177, "9") -> (w179:string)
      }
    }
    n87 = call "VerificarStop.vi"("error in"=w53, "Notifier in"=w52) -> ("stop"=w54:bool)  [unwired: 6 in, 2 out]
    n88 = local write "Password"(w58) -> ()
    n89 = call "LogError.vi"("Error In"=w57, "Path"=path "u:/logerrornotificacion.txt") -> ("Error Out"=w56:errorcluster)  [unwired: 8 in, 1 out]
  }
  n90 = while {
    tunnel: w26 -> [w193]
    tunnel: w26 -> [w191]
    tunnel: w31 -> [w190]
    tunnel: [w188] -> w32
    i -> [w181]
    stop <- w192 stop-if-true
    # "Sincronización HTTP POST"
    n91 = Quotient & Remainder(x=w181, y=60) -> (x-y*floor(x/y)=w186:i32)  [unwired: 1 out]
    n92 = Equal To 0?(x=w186) -> (x = 0?=w185:bool)
    n93 = Not Equal To 0?(x=w181) -> (x != 0?=w184:bool)
    n94 = And(x=w185, y=w184) -> (x .and. y?=w183:bool)
    n95 = case shown="True" w183 {
      tunnel: w193 -> [w194 w206]
      tunnel: [w194 w205] -> w189
      frame False {
      }
      frame True {
        n96 = call "FGV Semaforo.vi"("Function"=enum16{"GET", "SET"}."GET") -> ("semaphore out"=w200:T9)  [unwired: 10 in]
        n97 = call <vilib>:"Acquire Semaphore.vi"("error in (no error)"=w206, "semaphore"=w200) -> ("error out"=w196:errorcluster, "semaphore out"=w198:T9)  [unwired: 3 in, 1 out]
        n98 = call "CHECK SERVER CONECTION.vi"("error in (no error)"=w196, "semaphore"=w198) -> ("error out"=w195:errorcluster, "semaphore out"=w197:T9)  [unwired: 8 in]
        n99 = call "SincronizacionMain.vi"("max"=i64 100, "error in"=w195, "existe archivo"=TRUE, "semaphore"=w197) -> ("error out"=w204:errorcluster, "semaphore out"=w202:T9)  [unwired: 4 in, 2 out]
        n100 = call <vilib>:"Release Semaphore.vi"("error in (no error)"=w204, "semaphore"=w202) -> ("error out"=w205:errorcluster)  [unwired: 4 in, 1 out]
      }
    }
    n101 = call "VerificarStop.vi"("error in"=w191, "Notifier in"=w190) -> ("stop"=w192:bool)  [unwired: 6 in, 2 out]
    n102 = call "LogError.vi"("Error In"=w189, "Path"=path "u:/logerrorhttppost.txt") -> ("Error Out"=w188:errorcluster)  [unwired: 8 in, 1 out]
    n103 = Wait (ms)(milliseconds to wait=u32 1000) -> ()  [unwired: 1 out]
  }
  n104 = while {
    tunnel: w26 -> [w220]
    tunnel: w26 -> [w218]
    tunnel: w31 -> [w217]
    tunnel: [w207] -> w28
    i -> [w208]
    stop <- w219 stop-if-true
    # "Sincronizacion FTP"
    n105 = Quotient & Remainder(x=w208, y=100) -> (x-y*floor(x/y)=w212:i32)  [unwired: 1 out]
    n106 = Equal To 0?(x=w212) -> (x = 0?=w213:bool)
    n107 = Not Equal To 0?(x=w208) -> (x != 0?=w214:bool)
    n108 = And(x=w213, y=w214) -> (x .and. y?=w211:bool)
    n109 = case shown="True" w211 {
      tunnel: w220 -> [w221 w239]
      tunnel: [w221 w244] -> w215
      frame False {
      }
      frame True {
        n110 = call "FGV Semaforo.vi"("Function"=enum16{"GET", "SET"}."GET") -> ("semaphore out"=w228:T9)  [unwired: 10 in]
        n111 = call <vilib>:"Acquire Semaphore.vi"("error in (no error)"=w239, "semaphore"=w228) -> ("error out"=w225:errorcluster, "semaphore out"=w222:T9)  [unwired: 3 in, 1 out]
        n112 = call "CHECK SERVER CONECTION.vi"("error in (no error)"=w225, "semaphore"=w222) -> ("error out"=w224:errorcluster, "semaphore out"=w223:T9)  [unwired: 8 in]
        n113 = call "SincronizacionMain.vi"("max"=i64 360, "error in"=w224, "existe archivo"=TRUE, "semaphore"=w223) -> ("error out"=w233:errorcluster, "semaphore out"=w232:T9)  [unwired: 4 in, 2 out]
        n114 = call "FTP (SubVI).vi"("error in"=w233, "semaphore"=w232) -> ("error IO"=w227:errorcluster, "semaphore out"=w238:T9)  [unwired: 8 in]
        n115 = call "clearChannels.vi"("error in"=w227, "semaphore"=w238) -> ("error out"=w237:errorcluster, "semaphore out"=w236:T9)  [unwired: 8 in]
        n116 = call "registrarOffset.vi"("error in (no error)"=w237, "Offsets"=i64[] [0, 0, 0], "semaphore"=w236) -> ("error out"=w242:errorcluster, "semaphore out"=w235:T9)  [unwired: 7 in]
        n117 = call "ReduceRowsTDMS.vi"("Max Rows"=17000, "error in"=w242, "Array"=string[][] [["grupo1", "Radiacion"], ["grupo2", "I_load_Chr_Pnl_Sys"], ["grupo3", "Gen_VRMS"]], "semaphore"=w235) -> ("error out"=w241:errorcluster, "semaphore out"=w234:T9)  [unwired: 6 in]
        n118 = call <vilib>:"Release Semaphore.vi"("error in (no error)"=w241, "semaphore"=w234) -> ("error out"=w244:errorcluster)  [unwired: 4 in, 1 out]
      }
    }
    n119 = call "VerificarStop.vi"("error in"=w218, "Notifier in"=w217) -> ("stop"=w219:bool)  [unwired: 6 in, 2 out]
    n120 = Wait (ms)(milliseconds to wait=u32 1000) -> ()  [unwired: 1 out]
    n121 = call "LogError.vi"("Error In"=w215, "Path"=path "u:/logerrorftp.txt") -> ("Error Out"=w207:errorcluster)  [unwired: 8 in, 1 out]
  }
  n122 = while {
    tunnel: w31 -> [w246]
    tunnel: [w254] -> w37
    tunnel: [w250] -> w42
    tunnel: [w257] -> w41
    tunnel: [w256] -> w40
    tunnel: [w255] -> w39
    tunnel: w26 -> [w245]
    tunnel: [w252] -> w27
    tunnel: w11 -> [w248]
    stop <- w247 stop-if-true
    # "Ejecución Eventos"
    n123 = Get Notifier Status(notifier=w246, error in (no error)=w245) -> (notifier out=w258:refnum<notifier>, current notification=w260:T7, error out=w259:errorcluster)  [unwired: 2 out]
    n124 = case shown="\"Escribir\", Default" w260 {
      tunnel: w258 -> [w267 w293 w319 w332 w347 w359 w374 w387 w402 w417 w432 w447 w463 w481 w525]
      tunnel: w259 -> [w268 w294 w315 w325 w344 w356 w372 w386 w400 w415 w430 w445 w461 w483 w524]
      tunnel: [w268 w291 w313 w329 w345 w358 w370 w383 w401 w416 w431 w446 w464 w484 w526] -> w253
      tunnel: [w263 w271 w318 w322 w336 w350 w364 w378 w392 w407 w422 w437 w452 w476 w517] -> w257
      tunnel: [w262 w270 w317 w321 w335 w349 w363 w377 w391 w406 w421 w436 w451 w475 w516] -> w256
      tunnel: [w261 w269 w316 w320 w334 w348 w362 w376 w390 w405 w420 w435 w450 w474 w515] -> w255
      tunnel: [w267 w292 w319 w330 w342 w355 w366 w384 w398 w412 w427 w442 w458 w480 w527] -> w250
      tunnel: [w265 w289 w312 w328 w341 w353 w367 w380 w395 w410 w425 w441 w455 w478 w521] -> w252
      tunnel: w248 -> [w264 w272 w299 w323 w337 w351 w365 w379 w393 w408 w423 w438 w453 w477 w518]
      frame "Stop" {
        n125 = call "FGV Semaforo.vi"("Function"=enum16{"GET", "SET"}."GET") -> ("semaphore out"=w265:T9)  [unwired: 10 in]
        n126 = Unbundle(w264) -> ("queueM1 out"=w263:refnum<queue>, "queueM2 out"=w262:refnum<queue>, "queueM3 out"=w261:refnum<queue>)
      }
      frame "Iniciado" {
        w279 = T4 {"Left"=1050, "Top"=425} ("Position")
        w285 = T4 {"Left"=1300, "Top"=1120} ("Position")
        w286 = T4 {"Left"=1800, "Top"=1145} ("Position")
        w287 = T4 {"Left"=1000, "Top"=500} ("Position")
        w288 = T5 {"Width"=1000, "Height"=500} ("Plot Area:Size")
        n127 = property on="Graph Radiacion solar global" class="XYGraph (strict)"("Position"=w287) -> ()  [unwired: 2 in, 2 out]
        n128 = property on="XY Graph Temperatura" class="XYGraph (strict)"("Position"=w287) -> ()  [unwired: 2 in, 2 out]
        n129 = property on="XY Humedad Relativa" class="XYGraph (strict)"("Position"=w287) -> ()  [unwired: 2 in, 2 out]
        n130 = property on="XY Graph Temperatura de Panel" class="XYGraph (strict)"("Position"=w287) -> ()  [unwired: 2 in, 2 out]
        n131 = property on="XY Graph Potencia" class="XYGraph (strict)"("Position"=w287) -> ()  [unwired: 2 in, 2 out]
        n132 = property on="XY Graph Temperatura" class="XYGraph (strict)"("Plot Area Size"=w288) -> ()  [unwired: 2 in, 2 out]
        n133 = property on="XY Graph Radiacion solar global" class="XYGraph (strict)"("Plot Area Size"=w288) -> ()  [unwired: 2 in, 2 out]
        n134 = property on="XY Humedad Relativa" class="XYGraph (strict)"("Plot Area Size"=w288) -> ()  [unwired: 2 in, 2 out]
        n135 = property on="XY Graph Temperatura de Panel" class="XYGraph (strict)"("Plot Area Size"=w288) -> ()  [unwired: 2 in, 2 out]
        n136 = property on="XY Graph Potencia" class="XYGraph (strict)"("Plot Area Size"=w288) -> ()  [unwired: 2 in, 2 out]
        n137 = Send Notification(notification=EnumEstado."Escribir", notifier=w293, error in (no error)=w294) -> (notifier out=w292:refnum<notifier>, error out=w291:errorcluster)
        n138 = property on="XY Graph Potencia" class="XYGraph (strict)"("Position"=T4 {"Left"=1000, "Top"=480}) -> ()  [unwired: 2 in, 2 out]
        n139 = call "FGV Semaforo.vi"("Function"=enum16{"GET", "SET"}."GET") -> ("semaphore out"=w289:T9)  [unwired: 10 in]
        n140 = property on="Tab1_volver_tempambiente" class="Bool (strict)"("Position"=w286) -> ()  [unwired: 2 in, 2 out]
        n141 = property on="Tab1_volver_radiacion" class="Bool (strict)"("Position"=w286) -> ()  [unwired: 2 in, 2 out]
        n142 = property on="Tab1_volver_humedad" class="Bool (strict)"("Position"=w286) -> ()  [unwired: 2 in, 2 out]
        n143 = property on="Tab1_volver_potencia" class="Bool (strict)"("Position"=w286) -> ()  [unwired: 2 in, 2 out]
        n144 = property on="Tab1_volver_tempsuper" class="Bool (strict)"("Position"=w286) -> ()  [unwired: 2 in, 2 out]
        n145 = property on="Radiacion Tab 1" class="Bool"("Position"=w285) -> ()  [unwired: 2 in, 2 out]
        n146 = property on="Temperatura Tab 1" class="Bool"("Position"=w285) -> ()  [unwired: 2 in, 2 out]
        n147 = property on="Humedad Relativa Tab 1" class="Bool"("Position"=w285) -> ()  [unwired: 2 in, 2 out]
        n148 = property on="Temperatura de Panel Tab 1" class="Bool"("Position"=w285) -> ()  [unwired: 2 in, 2 out]
        n149 = Unbundle(w272) -> ("queueM1 out"=w271:refnum<queue>, "queueM2 out"=w270:refnum<queue>, "queueM3 out"=w269:refnum<queue>)
        n150 = property on="String 6" class="Str"("Position"=w279) -> ()  [unwired: 2 in, 2 out]
        n151 = property on="String 4" class="Str"("Position"=w279) -> ()  [unwired: 2 in, 2 out]
        n152 = property on="String 3" class="Str"("Position"=w279) -> ()  [unwired: 2 in, 2 out]
        n153 = property on="String 5" class="Str"("Position"=w279) -> ()  [unwired: 2 in, 2 out]
        n154 = property on="String 2" class="Str"("Position"=w279) -> ()  [unwired: 2 in, 2 out]
        "String 2" <- "RADIACION SOLAR GLOBAL ( w/m2 )"
        "String 3" <- "TEMPERATURA AMBIENTE  ( ° C )"
        "String 4" <- "HUMEDAD RELATIVA ( % )"
        "String 5" <- "TEMPERATURA DE PANEL ( ° C )"
        "String 6" <- "POTENCIA"
        "String 7" <- "CUADRO SINÓPTICO" ("String 7")
        "String 8" <- "PANEL FOTOVOLTAICO (kW)" ("String 8")
        "String 9" <- "NIVEL DE BATERIA (%)" ("String 9")
        "String 10" <- "CARGA (kW)" ("String 10")
        "String 11" <- "GENERADOR (kW)" ("String 11")
      }
      frame "Escribir", Default {
        n155 = call "FGV Semaforo.vi"("Function"=enum16{"GET", "SET"}."GET") -> ("semaphore out"=w304:T9)  [unwired: 10 in]
        n156 = Unbundle(w299) -> ("queueM1 out"=w298:refnum<queue>, "queueM2 out"=w296:refnum<queue>, "queueM3 out"=w297:refnum<queue>)
        n157 = call <vilib>:"Acquire Semaphore.vi"("error in (no error)"=w315, "semaphore"=w304) -> ("error out"=w314:errorcluster, "semaphore out"=w311:T9)  [unwired: 3 in, 1 out]
        n158 = call "Escribir TDMS Parametro Meteorologico.vi"("semaphore"=w311, "error in"=w314, "queue"=w298) -> ("error out"=w307:errorcluster, "queue out"=w318:refnum<queue>, "semaphore out"=w310:T9)  [unwired: 4 in, 2 out]
        n159 = call "Escribir TDMS Parametro del Generador.vi"("semaphore"=w310, "queue"=w297) -> ("error out"=w308:errorcluster, "queue out"=w317:refnum<queue>, "semaphore out"=w309:T9)  [unwired: 5 in, 2 out]
        n160 = call "Escribir TDMS Parametros Inversor.vi"("semaphore"=w309, "queue"=w296) -> ("error out"=w306:errorcluster, "queue out"=w316:refnum<queue>, "semaphore out"=w302:T9)  [unwired: 5 in, 2 out]
        n161 = Merge Errors(w306, w308, w307) -> (w303:errorcluster)
        n162 = call "Eliminar TDMS.vi"("error in"=w303, "semaphore"=w302) -> ("error out"=w300:errorcluster, "semaphore out"=w301:T9)  [unwired: 8 in]
        n163 = call <vilib>:"Release Semaphore.vi"("error in (no error)"=w300, "semaphore"=w301) -> ("error out"=w313:errorcluster, "semaphore out"=w312:T9)  [unwired: 4 in]
      }
      frame "Leer Radiacion" {
        n164 = call "Graficar.vi"("error in"=w325, "group name"="grupo1", "channel name"="Radiacion") -> ("error out"=w331:errorcluster, "XY Graph"=→"Radiacion solar global":cluster{timestamp[], dbl[]}, "semaphore out"=w328:T9)  [unwired: 6 in]
        n165 = Send Notification(notification=EnumEstado."Escribir", notifier=w332, error in (no error)=w331) -> (notifier out=w330:refnum<notifier>, error out=w329:errorcluster)
        n166 = Unbundle(w323) -> ("queueM1 out"=w322:refnum<queue>, "queueM2 out"=w321:refnum<queue>, "queueM3 out"=w320:refnum<queue>)
      }
      frame "Leer Temp" {
        n167 = call "Graficar.vi"("error in"=w344, "group name"="grupo1", "channel name"="Temp ambiente") -> ("error out"=w343:errorcluster, "XY Graph"=→"XY Graph Temperatura":cluster{timestamp[], dbl[]}, "semaphore out"=w341:T9)  [unwired: 6 in]
        n168 = Send Notification(notification=EnumEstado."Escribir", notifier=w347, error in (no error)=w343) -> (notifier out=w342:refnum<notifier>, error out=w345:errorcluster)
        n169 = Unbundle(w337) -> ("queueM1 out"=w336:refnum<queue>, "queueM2 out"=w335:refnum<queue>, "queueM3 out"=w334:refnum<queue>)
      }
      frame "Leer Humed Relat" {
        n170 = call "Graficar.vi"("error in"=w356, "group name"="grupo1", "channel name"="Humedad Relat") -> ("error out"=w357:errorcluster, "XY Graph"=→"XY Humedad Relativa":cluster{timestamp[], dbl[]}, "semaphore out"=w353:T9)  [unwired: 6 in]
        n171 = Send Notification(notification=EnumEstado."Escribir", notifier=w359, error in (no error)=w357) -> (notifier out=w355:refnum<notifier>, error out=w358:errorcluster)
        n172 = Unbundle(w351) -> ("queueM1 out"=w350:refnum<queue>, "queueM2 out"=w349:refnum<queue>, "queueM3 out"=w348:refnum<queue>)
      }
      frame "Leer Temp del Panel" {
        n173 = call "Graficar.vi"("error in"=w372, "group name"="grupo1", "channel name"="Temp panel") -> ("error out"=w371:errorcluster, "XY Graph"=→"XY Graph Temperatura de Panel":cluster{timestamp[], dbl[]}, "semaphore out"=w367:T9)  [unwired: 6 in]
        n174 = Send Notification(notification=EnumEstado."Escribir", notifier=w374, error in (no error)=w371) -> (notifier out=w366:refnum<notifier>, error out=w370:errorcluster)
        n175 = Unbundle(w365) -> ("queueM1 out"=w364:refnum<queue>, "queueM2 out"=w363:refnum<queue>, "queueM3 out"=w362:refnum<queue>)
      }
      frame "Leer Pot Panel" {
        n176 = call "Graficar.vi"("error in"=w386, "group name"="grupo2", "channel name"="Pot_Panel") -> ("error out"=w385:errorcluster, "XY Graph"=→"XY Graph Potencia":cluster{timestamp[], dbl[]}, "semaphore out"=w380:T9)  [unwired: 6 in]
        n177 = Send Notification(notification=EnumEstado."Escribir", notifier=w387, error in (no error)=w385) -> (notifier out=w384:refnum<notifier>, error out=w383:errorcluster)
        n178 = Unbundle(w379) -> ("queueM1 out"=w378:refnum<queue>, "queueM2 out"=w377:refnum<queue>, "queueM3 out"=w376:refnum<queue>)
      }
      frame "Leer Pot Fase R" {
        n179 = call "Graficar.vi"("error in"=w400, "group name"="grupo2", "channel name"="Pot_load_R") -> ("error out"=w399:errorcluster, "XY Graph"=w394:cluster{timestamp[], dbl[]}, "semaphore out"=w395:T9)  [unwired: 6 in]
        n180 = property on="XY Graph Potencia" class="XYGraph (strict)"(error in=w399, "Val(Sgnl)"=w394) -> (error out=w397:errorcluster)  [unwired: 1 in, 1 out]
        n181 = Send Notification(notification=EnumEstado."Escribir", notifier=w402, error in (no error)=w397) -> (notifier out=w398:refnum<notifier>, error out=w401:errorcluster)
        n182 = Unbundle(w393) -> ("queueM1 out"=w392:refnum<queue>, "queueM2 out"=w391:refnum<queue>, "queueM3 out"=w390:refnum<queue>)
      }
      frame "Leer Pot Fase  S" {
        n183 = call "Graficar.vi"("error in"=w415, "group name"="grupo2", "channel name"="Pot_load_S") -> ("error out"=w414:errorcluster, "XY Graph"=w409:cluster{timestamp[], dbl[]}, "semaphore out"=w410:T9)  [unwired: 6 in]
        n184 = property on="XY Graph Potencia" class="XYGraph (strict)"(error in=w414, "Val(Sgnl)"=w409) -> (error out=w413:errorcluster)  [unwired: 1 in, 1 out]
        n185 = Send Notification(notification=EnumEstado."Escribir", notifier=w417, error in (no error)=w413) -> (notifier out=w412:refnum<notifier>, error out=w416:errorcluster)
        n186 = Unbundle(w408) -> ("queueM1 out"=w407:refnum<queue>, "queueM2 out"=w406:refnum<queue>, "queueM3 out"=w405:refnum<queue>)
      }
      frame "Leer PotFase T" {
        n187 = call "Graficar.vi"("error in"=w430, "group name"="grupo2", "channel name"="Pot_load_T") -> ("error out"=w429:errorcluster, "XY Graph"=w424:cluster{timestamp[], dbl[]}, "semaphore out"=w425:T9)  [unwired: 6 in]
        n188 = property on="XY Graph Potencia" class="XYGraph (strict)"(error in=w429, "Val(Sgnl)"=w424) -> (error out=w428:errorcluster)  [unwired: 1 in, 1 out]
        n189 = Send Notification(notification=EnumEstado."Escribir", notifier=w432, error in (no error)=w428) -> (notifier out=w427:refnum<notifier>, error out=w431:errorcluster)
        n190 = Unbundle(w423) -> ("queueM1 out"=w422:refnum<queue>, "queueM2 out"=w421:refnum<queue>, "queueM3 out"=w420:refnum<queue>)
      }
      frame "Leer Pot Generador" {
        n191 = call "Graficar.vi"("error in"=w445, "group name"="grupo3", "channel name"="Gen_KW") -> ("error out"=w444:errorcluster, "XY Graph"=w440:cluster{timestamp[], dbl[]}, "semaphore out"=w441:T9)  [unwired: 6 in]
        n192 = property on="XY Graph Potencia" class="XYGraph (strict)"(error in=w444, "Val(Sgnl)"=w440) -> (error out=w443:errorcluster)  [unwired: 1 in, 1 out]
        n193 = Send Notification(notification=EnumEstado."Escribir", notifier=w447, error in (no error)=w443) -> (notifier out=w442:refnum<notifier>, error out=w446:errorcluster)
        n194 = Unbundle(w438) -> ("queueM1 out"=w437:refnum<queue>, "queueM2 out"=w436:refnum<queue>, "queueM3 out"=w435:refnum<queue>)
      }
      frame "Leer Nivel Bat" {
        n195 = call "Graficar.vi"("error in"=w461, "group name"="grupo2", "channel name"="Pot_bat") -> ("error out"=w460:errorcluster, "XY Graph"=w454:cluster{timestamp[], dbl[]}, "semaphore out"=w455:T9)  [unwired: 6 in]
        n196 = property on="XY Graph Potencia" class="XYGraph (strict)"(error in=w460, "Val(Sgnl)"=w454) -> (error out=w459:errorcluster)  [unwired: 1 in, 1 out]
        n197 = Send Notification(notification=EnumEstado."Escribir", notifier=w463, error in (no error)=w459) -> (notifier out=w458:refnum<notifier>, error out=w464:errorcluster)
        n198 = Unbundle(w453) -> ("queueM1 out"=w452:refnum<queue>, "queueM2 out"=w451:refnum<queue>, "queueM3 out"=w450:refnum<queue>)
      }
      frame "Log In" {
        n199 = Open/Create/Replace File(file path (use dialog)=path "u:/login/login.txt", operation (0:open)=T10."open") -> (refnum out=w469:refnum<file>, error out=w473:errorcluster)  [unwired: 4 in, 1 out]
        n200 = Read from Text File(file (use dialog)=w469, error in=w473) -> (refnum out=w468:refnum<file>, text=w467:string, error out=w472:errorcluster)  [unwired: 2 in, 1 out]
        n201 = Close File(refnum=w468, error in=w472) -> ()  [unwired: 2 out]
        n202 = Equal?(x=w467, y="Password") -> (x = y?=w485:bool)
        n203 = case shown="False" w485 {
          tunnel: [w497 w508] -> w482
          tunnel: w483 -> [w496 w510]
          tunnel: [w493 EnumEstado."Escribir" ("notification")] -> w466
          tunnel: "Password" -> [w494 _]
          frame False {
            n204 = Open/Create/Replace File(file path (use dialog)=path "u:/login/logout.txt", operation (0:open)=T10."open") -> (refnum out=w491:refnum<file>, error out=w487:errorcluster)  [unwired: 4 in, 1 out]
            n205 = Read from Text File(file (use dialog)=w491, error in=w487) -> (refnum out=w492:refnum<file>, text=w486:string, error out=w488:errorcluster)  [unwired: 2 in, 1 out]
            n206 = Equal?(x=w494, y=w486) -> (x = y?=w495:bool)
            n207 = Close File(refnum=w492, error in=w488) -> ()  [unwired: 2 out]
            n208 = case shown="True" w495 {
              tunnel: ["Password Incorrecto" ("String") "Deteniendo..." ("String")] -> w498
              tunnel: [EnumEstado."Escribir" ("notification") EnumEstado."Stop" ("notification")] -> w493
              tunnel: [w499 w503] -> w497
              tunnel: w496 -> [w499 w503]
              frame False {
              }
              frame True {
              }
            }
            "String" <- w498
          }
          frame True {
            n209 = property on="Tab Control 2" class="TabCtl (strict)"(error in=w510, "Visible"=FALSE) -> (error out=w512:errorcluster)  [unwired: 1 in, 1 out]
            n210 = property on="String" class="Str"("Text.Text"="") -> ()  [unwired: 2 in, 2 out]
            n211 = property on="Tab Control" class="TabCtl (strict)"(error in=w512, "Visible"=TRUE) -> (error out=w509:errorcluster)  [unwired: 1 in, 1 out]
            n212 = property on="logout" class="Bool (strict)"(error in=w509, "Visible"=TRUE) -> (error out=w508:errorcluster)  [unwired: 1 in, 1 out]
          }
        }
        n213 = call "FGV Semaforo.vi"("Function"=enum16{"GET", "SET"}."GET") -> ("semaphore out"=w478:T9)  [unwired: 10 in]
        n214 = Send Notification(notification=w466, notifier=w481, error in (no error)=w482) -> (notifier out=w480:refnum<notifier>, error out=w484:errorcluster)
        n215 = Unbundle(w477) -> ("queueM1 out"=w476:refnum<queue>, "queueM2 out"=w475:refnum<queue>, "queueM3 out"=w474:refnum<queue>)
      }
      frame "Log Out" {
        n216 = property on="Tab Control 2" class="TabCtl (strict)"(error in=w524, "Visible"=TRUE) -> (error out=w530:errorcluster)  [unwired: 1 in, 1 out]
        n217 = property on="Tab Control" class="TabCtl (strict)"(error in=w530, "Visible"=FALSE) -> (error out=w520:errorcluster)  [unwired: 1 in, 1 out]
        n218 = property on="logout" class="Bool (strict)"(error in=w520, "Visible"=FALSE) -> (error out=w519:errorcluster)  [unwired: 1 in, 1 out]
        n219 = Send Notification(notification=EnumEstado."Escribir", notifier=w525, error in (no error)=w519) -> (notifier out=w527:refnum<notifier>, error out=w526:errorcluster)
        n220 = call "FGV Semaforo.vi"("Function"=enum16{"GET", "SET"}."GET") -> ("semaphore out"=w521:T9)  [unwired: 10 in]
        n221 = Unbundle(w518) -> ("queueM1 out"=w517:refnum<queue>, "queueM2 out"=w516:refnum<queue>, "queueM3 out"=w515:refnum<queue>)
      }
    }
    n222 = call "VerificarStop.vi"("error in"=w245, "Notifier in"=w246) -> ("stop"=w247:bool)  [unwired: 6 in, 2 out]
    n223 = Wait (ms)(milliseconds to wait=u32 200) -> ()  [unwired: 1 out]
    n224 = call "LogError.vi"("Error In"=w253, "Path"=path "u:/logerroreventos.txt") -> ("Error Out"=w254:errorcluster)  [unwired: 8 in, 1 out]
  }
  n225 = while {
    tunnel: w26 -> [w584]
    tunnel: [w574] -> w38
    tunnel: [w593] -> w48
    tunnel: w26 -> [w592]
    tunnel: [w591] -> w47
    tunnel: w31 -> [w589]
    tunnel: w26 -> [w588]
    tunnel: refnum<visa-resource-name> "ASRL2::INSTR" ("VISA resource name") -> [w575]
    tunnel: w26 -> [w548]
    tunnel: w11 -> [w542]
    stop <- w590 stop-if-true
    # "Bypass = 0"
    # "Pot_gen > 0"
    # "Adquisición de Parámetros Meteorológicos, del Inversor y Generador"
    n226 = Unbundle(w542) -> ("queueM1 out"=w541:refnum<queue>, "queueM2 out"=w540:refnum<queue>, "queueM3 out"=w539:refnum<queue>)
    n227 = call "Adquirir Parametro Inversor por SNMP.vi"("queue in"=w540, "error in"=w584) -> ("result"=w559:dbl[], "Flujo_Bypass"=w531:bool, "Time inversor"=→"ÚLTIMA MEDICIÓN DEL \nINVERSOR":timestamp, "Flujo_Bat_Carga"=→"Flujo_Bat_carg":bool, "Flujo_Bat_Descarga"=→"Flujo_Bat_descarga":bool, "Flujo_Panel"=→"Flujo_Panel":bool, "Flujo_Load"=w535:bool, "Pot_Panel_Out"=→"valor_panel":dbl, "Pot_Load_Out"=→"valor_carga":dbl, "Nivel_bat_Out"=→"valor_bateria":dbl, "Ring_Panel_Out"=→"Ring_Panel":i32, "error de conexion"=w532:bool, "Ring_Nivel_Bat_Out"=→"Ring_Nivel_bat":i32, "Ring_Inversor_Out"=→"Ring_Inversor":i32, "error out"=w583:errorcluster)  [unwired: 11 in]
    "Flujo_Load" <- w535
    "Flujo_Bypass" <- w531
    n228 = call "Adquirir Parametro Meteorologico.vi"("error in"=w548, "queue in"=w541) -> ("error out"=w547:errorcluster)  [unwired: 8 in, 1 out]
    n229 = Not(x=w531) -> (.not. x?=w537:bool)
    n230 = call "Adquirir Parametro del Generador por Modbus.vi"("error in"=w592, "VISA resource name"=w575, "queue"=w539) -> ("error out"=w587:errorcluster, "Ring_Gen_Out"=→"Ring_Gen":i32, "Pot_gen_out"=→"valor_generador":dbl, "Time_gen"=→"ÚLTIMA MEDICIÓN DEL\n G. DIESEL":timestamp, "Flujo_Gen_Out"=w538:bool)  [unwired: 3 in, 1 out]
    n231 = And(x=w538, y=w537) -> (x .and. y?=w534:bool)
    "Flujo_Gen" <- w534
    n232 = case shown="True" w532 {
      tunnel: w535 -> [w597 _]
      tunnel: w534 -> [w596 _]
      tunnel: [w594 2] -> w533
      frame False {
        n233 = Or(x=w597, y=w596) -> (x .or. y?=w595:bool)
        n234 = case shown="False" w595 {
          tunnel: [1 0] -> w594
          frame False {
          }
          frame True {
          }
        }
      }
      frame True {
      }
    }
    "Ring_Load" <- w533
    n235 = call "VerificarStop.vi"("error in"=w588, "Notifier in"=w589) -> ("stop"=w590:bool)  [unwired: 6 in, 2 out]
    n236 = call "LogError.vi"("Error In"=w547, "Path"=path "u:/logerrormeteorologico.txt") -> ("Error Out"=w574:errorcluster)  [unwired: 8 in, 1 out]
    n237 = Index Array(array=w559, index #1=14 ("index"), index #2=15 ("index"), index #3=16 ("index"), index #4=17 ("index"), index #5=18 ("index"), index #6=19 ("index"), index #7=20 ("index")) -> (element #1=w567:dbl, element #2=w568:dbl, element #3=w569:dbl, element #4=w570:dbl, element #5=w571:dbl, element #6=w572:dbl, element #7=w573:dbl)
    n238 = Greater Than 0?(x=w568) -> (x > 0?=w558:bool)
    "Falla monofásica" <- w558
    n239 = Greater Than 0?(x=w569) -> (x > 0?=w557:bool)
    "Falla trifásica" <- w557
    n240 = Greater Than 0?(x=w570) -> (x > 0?=w556:bool)
    "Nivel de batería baja" <- w556
    n241 = Greater Than 0?(x=w571) -> (x > 0?=w555:bool)
    "Falla nivel de batería alta" <- w555
    n242 = Greater Than 0?(x=w572) -> (x > 0?=w554:bool)
    "Falla en módulo" <- w554
    n243 = Greater Than 0?(x=w573) -> (x > 0?=w553:bool)
    "Alta temperatura\n en gabinete" <- w553
    n244 = Greater Than 0?(x=w567) -> (x > 0?=w552:bool)
    "Algun mal funcionamiento \nen el SGH" <- w552
    n245 = call "LogError.vi"("Error In"=w583, "Path"=path "u:/logerrorinversor.txt") -> ("Error Out"=w593:errorcluster)  [unwired: 8 in, 1 out]
    n246 = call "LogError.vi"("Error In"=w587, "Path"=path "u:/logerrorgenerador.txt") -> ("Error Out"=w591:errorcluster)  [unwired: 8 in, 1 out]
    n247 = property on="Algun mal funcionamiento \nen el SGH" class="Bool (strict)"("Caption.Visible"=w552) -> ()  [unwired: 2 in, 2 out]
    n248 = property on="Falla monofásica" class="Bool (strict)"("Caption.Visible"=w558) -> ()  [unwired: 2 in, 2 out]
    n249 = property on="Falla trifásica" class="Bool (strict)"("Caption.Visible"=w557) -> ()  [unwired: 2 in, 2 out]
    n250 = property on="Nivel de batería baja" class="Bool (strict)"("Caption.Visible"=w556) -> ()  [unwired: 2 in, 2 out]
    n251 = property on="Falla nivel de batería alta" class="Bool (strict)"("Caption.Visible"=w555) -> ()  [unwired: 2 in, 2 out]
    n252 = property on="Falla en módulo" class="Bool (strict)"("Caption.Visible"=w554) -> ()  [unwired: 2 in, 2 out]
    n253 = property on="Alta temperatura\n en gabinete" class="Bool (strict)"("Caption.Visible"=w553) -> ()  [unwired: 2 in, 2 out]
    n254 = Wait (ms)(milliseconds to wait=u32 15000) -> ()  [unwired: 1 out]
  }
  n255 = Merge Errors(w28, w32, w36, w37, w38, w48, w47) -> (w46:errorcluster)
  n256 = Release Queue(queue=w41, error in (no error)=w46) -> (error out=w50:errorcluster)  [unwired: 1 in, 2 out]
  n257 = Release Queue(queue=w39, error in (no error)=w46) -> (error out=w45:errorcluster)  [unwired: 1 in, 2 out]
  n258 = Release Queue(queue=w40, error in (no error)=w46) -> (error out=w49:errorcluster)  [unwired: 1 in, 2 out]
  n259 = Merge Errors(w50, w49, w45) -> (w25:errorcluster)
  n260 = Release Notifier(notifier=w42, error in (no error)=w25) -> (error out=w7:errorcluster)  [unwired: 1 in, 2 out]
  n261 = call "FGV_FILE_PATH.vi"("Function"=enum16{"GET", "SET"}."GET") -> ("Data Out"=w9:T11)  [unwired: 10 in]
  n262 = Unbundle(w9) -> ("tdms control out"=w4:refnum<k34>, "tdms historial out"=w2:refnum<k34>, "tdms sinc out"=w1:refnum<k34>)
  n263 = TDMS Flush(4:w7, 7:w4) -> (0:w6:errorcluster, 3:w3:refnum<k34>)
  n264 = TDMS Close(8:w6, 11:w3) -> (0:w5:errorcluster)  [unwired: 1 out]
  n265 = TDMS Flush(4:w5, 7:w2) -> (0:w43:errorcluster, 3:w8:refnum<k34>)
  n266 = TDMS Close(8:w43, 11:w8) -> (0:w33:errorcluster)  [unwired: 1 out]
  n267 = TDMS Flush(4:w33, 7:w1) -> (0:w34:errorcluster, 3:w35:refnum<k34>)
  n268 = TDMS Close(8:w34, 11:w35) -> (0:w29:errorcluster)  [unwired: 1 out]
  n269 = call <vilib>:"Release Semaphore Reference.vi"("error in (no error)"=w29, "semaphore"=w27) -> ()  [unwired: 8 in, 2 out]
